vi "nanomachining test temperature.vi"() -> ()   [LabVIEW 2017]
uses:
  <vilib>/DAQmx/write.llb/DAQmx Write (Digital Bool 1Line 1Point).vi
  <vilib>/DAQmx/read.llb/DAQmx Read (Analog 1D DBL NChan 1Samp).vi
  <vilib>/DAQmx/create/channels.llb/DAQmx Create Channel (AI-Voltage-Basic).vi
  <vilib>/DAQmx/create/channels.llb/DAQmx Create Channel (DO-Digital Output).vi
  <vilib>/DAQmx/miscellaneous.llb/DAQmx Fill In Error Info.vi
  <vilib>/DAQmx/create/channels.llb/DAQmx Create Channel (AO-Voltage-Basic).vi
  <vilib>/Utility/file.llb/Write Delimited Spreadsheet (DBL).vi
  <vilib>/imath/engines/lvmath2/RunTimeEngine/Managers/WorkSpace/UID Generator.vi
  <vilib>/imath/engines/lvmath2/RunTimeEngine/RunTimeType/NIMS_RunTimeType_From StrictType (excl LVString).vi
  <instcachedir>/0/NIMS_RunTimeType_From StrictType (excl LVString)_1019F277F0A747EDBCA0F6C52CA54500.lvgen/NIMS_RunTimeType_From StrictType (excl LVString)_1019F277F0A747EDBCA0F6C52CA54500_000.vi
  <vilib>/imath/engines/lvmath2/RunTimeEngine/LocalVariableDefStatement/MC_LocalVariableDefStatement_Display.vi
  <vilib>/imath/engines/lvmath2/RunTimeEngine/Managers/SymbolTable/Clear UID.vi
  <vilib>/imath/engines/lvmath2/RunTimeEngine/NodeEndStatement/NIMS_NodeEndStatement_Output.vi
  <instcachedir>/0/NIMS_NodeEndStatement_Output_53EC0D466D134D7ABD903AC30B43404B.lvgen/NIMS_NodeEndStatement_Output_53EC0D466D134D7ABD903AC30B43404B_009.vi
  <vilib>/imath/engines/lvmath2/RunTimeEngine/ErrorHandling/NIMS_Finalize Error.vi
  <vilib>/imath/engines/lvmath2/RunTimeEngine/Managers/SymbolTable/NIMS_WorkSpace.lvlib
panel:
  in  "Stop Temperature Acquisition":bool
  in  "Pre exposure park time (msec)":u32=5000
  out "Y Park":dbl[](array[numeric])
  out "X Park":dbl[](array[numeric])
  out "Iterations areas 3":i32[](array[numeric])
  in  "Y Park (V)":dbl=10.0
  in  "X Park (V)":dbl=10.0
  in  "End exposure park time (msec)":u32=10000
  in  "Feature source file location":path
  in  "Scan Subvi-Back and Forth ?":bool
  in  "Start wait (msec)":u32=5000
  out "thermocouples (C)":dbl[](array[numeric])
  in  "Start test?":bool
  in  "Temperature control":bool
  in  "Test type":T1(tab)
  in  "Time for each line":dbl[](array[numeric])=[0.01, 0.0316, 0.1, 0.316, 1.0, 3.16, 10.0, 31.62, 100.0]
  in  "Iterations":u32=1
  in  "Line boundaries":dbl[](array[numeric])=[10.0, -10.0]
  in  "Lines position":dbl[](array[numeric])=[9.0, 8.0, 7.0, 6.0, 4.0, 1.5, -1.5, -5.0, -9.0]
  in  "Dwell time multiplication factor":dbl=1.0
  in  "Orientation":enum16{"Horizontal", "Vertical"}(ring)
  out "Lines done?":bool
  out "Iterations Lines":i32[](array[numeric])
  out "Exposure time":dbl[](array[numeric])
  out "Exposure time plus dwell time":dbl[](array[numeric])
  out "Lines done? 2":bool
  in  "Iterations 3":u32=1
  out "Exposure time 2":dbl[](array[numeric])
  out "Iterations Lines 2":i32[](array[numeric])
  out "Exposure time plus dwell time 2":dbl[](array[numeric])
  in  "Orientation 2":enum16{"Horizontal", "Vertical"}(ring)=enum."Vertical"
  in  "Dwell multiplication factor":dbl=1.0
  out "Time (sec)":dbl[](array[numeric])
  out "X (end) (V)":dbl[](array[numeric])
  out "Y (start) (V)":dbl[](array[numeric])
  out "X start (V)":dbl[](array[numeric])
  out "Y end (V)":dbl[](array[numeric])
  out "No. Pixels X":dbl[](array[numeric])
  out "No. Pixels Y":dbl[](array[numeric])
  out "Points done?":bool
  in  "Multiplicator for each instance":dbl[](array[numeric])=[0.01, 0.0316, 0.1, 0.316, 1.0, 3.16, 10.0, 31.6, 100.0]
  in  "Dwell time X factor":dbl=1.0
  in  "points X dup":dbl[](array[numeric])=[9.0, 6.0, 2.0, -3.0, -9.0, 7.5, 4.0, -0.5, -6.0]
  in  "points Y dup":dbl[](array[numeric])=[8.0, 8.0, 8.0, 8.0, 8.0, 3.0, 3.0, 3.0, 3.0]
  out "Elapsed times pointds":dbl[](array[numeric])
  out "Iterations points":i32[](array[numeric])
  out "el times 2 points":dbl[](array[numeric])
  in  "Times (s)":dbl[](array[numeric])=[0.53, 0.95, 1.69, 3.0, 5.33, 9.49, 16.87, 30.0, 53.35, 94.87, 168.7, 300.0]
  in  "Voltages y":dbl[][](array[numeric])=[[10.0, 6.0], [10.0, 6.0], [10.0, 6.0], [10.0, 6.0], [2.0, -2.0], [2.0, -2.0], [2.0, -2.0], [2.0, -2.0], [-6.0, -10.0], [-6.0, -10.0], [-6.0, -10.0], [-6.0, -10.0]]
  in  "Voltages x":dbl[][](array[numeric])=[[10.0, 7.0], [4.33, 1.33], [-1.33, -4.33], [-7.0, -10.0], [10.0, 7.0], [4.33, 1.33], [-1.33, -4.33], [-7.0, -10.0], [10.0, 7.0], [4.33, 1.33], [-1.33, -4.33], [-7.0, -10.0]]
  out "Elapsed times areas":dbl[](array[numeric])
  out "Iterations areas":i32[](array[numeric])
  out "El times areas 2":dbl[](array[numeric])
  out "Areas done?":bool
  in  "Mode":enum16{"Vertical", "Zigzag", "Horizontal"}(ring)
  in  "Freq":dbl=100000.0
  out "Elapsed Time (s)":dbl
  out "proj time":dbl
  out "Intensity Graph":dbl[][](graph)
  out "Iterations 2":i32
  in  "maxdepth":dbl=1.5
  in  "y range":dbl[](array[numeric])
  in  "x range":dbl[](array[numeric])
  in  "y pixels 2":dbl=100.0
  in  "x pixels 2":dbl=100.0
  in  "Frequency":dbl=100000.0
  out "Progress":dbl(slide) scale=0.0..1.0
  out "Dots done?":bool
  in  "Dwell time multiplicator":dbl=1.0
  out "Elapsed times points":dbl[](array[numeric])
  out "Iterations points 2":i32[](array[numeric])
  out "Loop Times points":dbl[](array[numeric])
  out "X start dots (V)":dbl[](array[numeric])
  out "Time (sec) 3":dbl[](array[numeric])
  out "Y start dots (V)":dbl[](array[numeric])
  in  "point mock frequency":dbl=10000.0 format="%#_13g"
  out "Elapsed times areas 2":dbl[](array[numeric])
  out "El times areas 3":dbl[](array[numeric])
  out "Iterations areas 2":i32[](array[numeric])
  in  "Stop Button 2":bool
  in  "Mode 2":enum16{"Vertical", "Zigzag", "Horizontal"}(ring)
  out "Line done?":bool
  in  "Dwell multiplication factor 2":dbl=0.5
  out "Time (sec) 2":dbl[](array[numeric])
  out "No. Pixels X 2":dbl[](array[numeric])
  out "No. Pixels Y 2":dbl[](array[numeric])
  out "X start (V) 2":dbl[](array[numeric])
  out "X (end) (V) 2":dbl[](array[numeric])
  out "Y (start) (V) 2":dbl[](array[numeric])
  out "Y end (V) 2":dbl[](array[numeric])
  in  "Freq 2":dbl=100000.0
  in  "Waveform Frequency":dbl=1000000.0
  in  "Area scan mode (Zigzag best)":enum16{"Vertical", "Zigzag", "Horizontal"}(ring)=enum."Zigzag"
  out "Areas done?":bool
  out "Frame Number":i32[](array[numeric])
  out "El times areas 4":dbl[](array[numeric])
  out "Elapsed times areas 3":dbl[](array[numeric])
  out "Time (s)":dbl[](array[numeric])
  in  "Dwell multiplication factor":dbl=1.0
  out "X start (V)":dbl[](array[numeric])
  out "X (end) (V)":dbl[](array[numeric])
  out "Y (start) (V)":dbl[](array[numeric])
  out "Y end (V)":dbl[](array[numeric])
  out "No. Pixels X":dbl[](array[numeric])
  out "Writing time (s)":dbl[](array[numeric])
  out "Corner dwell time (s)":dbl[](array[numeric])
  out "No. Pixels Y":dbl[](array[numeric])
  out "Autovoltage (V)":dbl
  out "thermocouples (V)":dbl[](array[numeric]) format="%0.4f"
  in  "Setpoint":dbl
  in  "Manual voltage (V)":dbl
  out "setpoint in mv":dbl
  out "I measured source":dbl format="%.2p"
  out "V source measured":dbl format="%.2p"
  out "Waveform Chart":cluster{dbl, dbl}(graph)
  in  "manual Temp. ?":bool
  in  "folder path":path
  # "automatically creates a copy on the bottom half of the screen ( negative Y)"
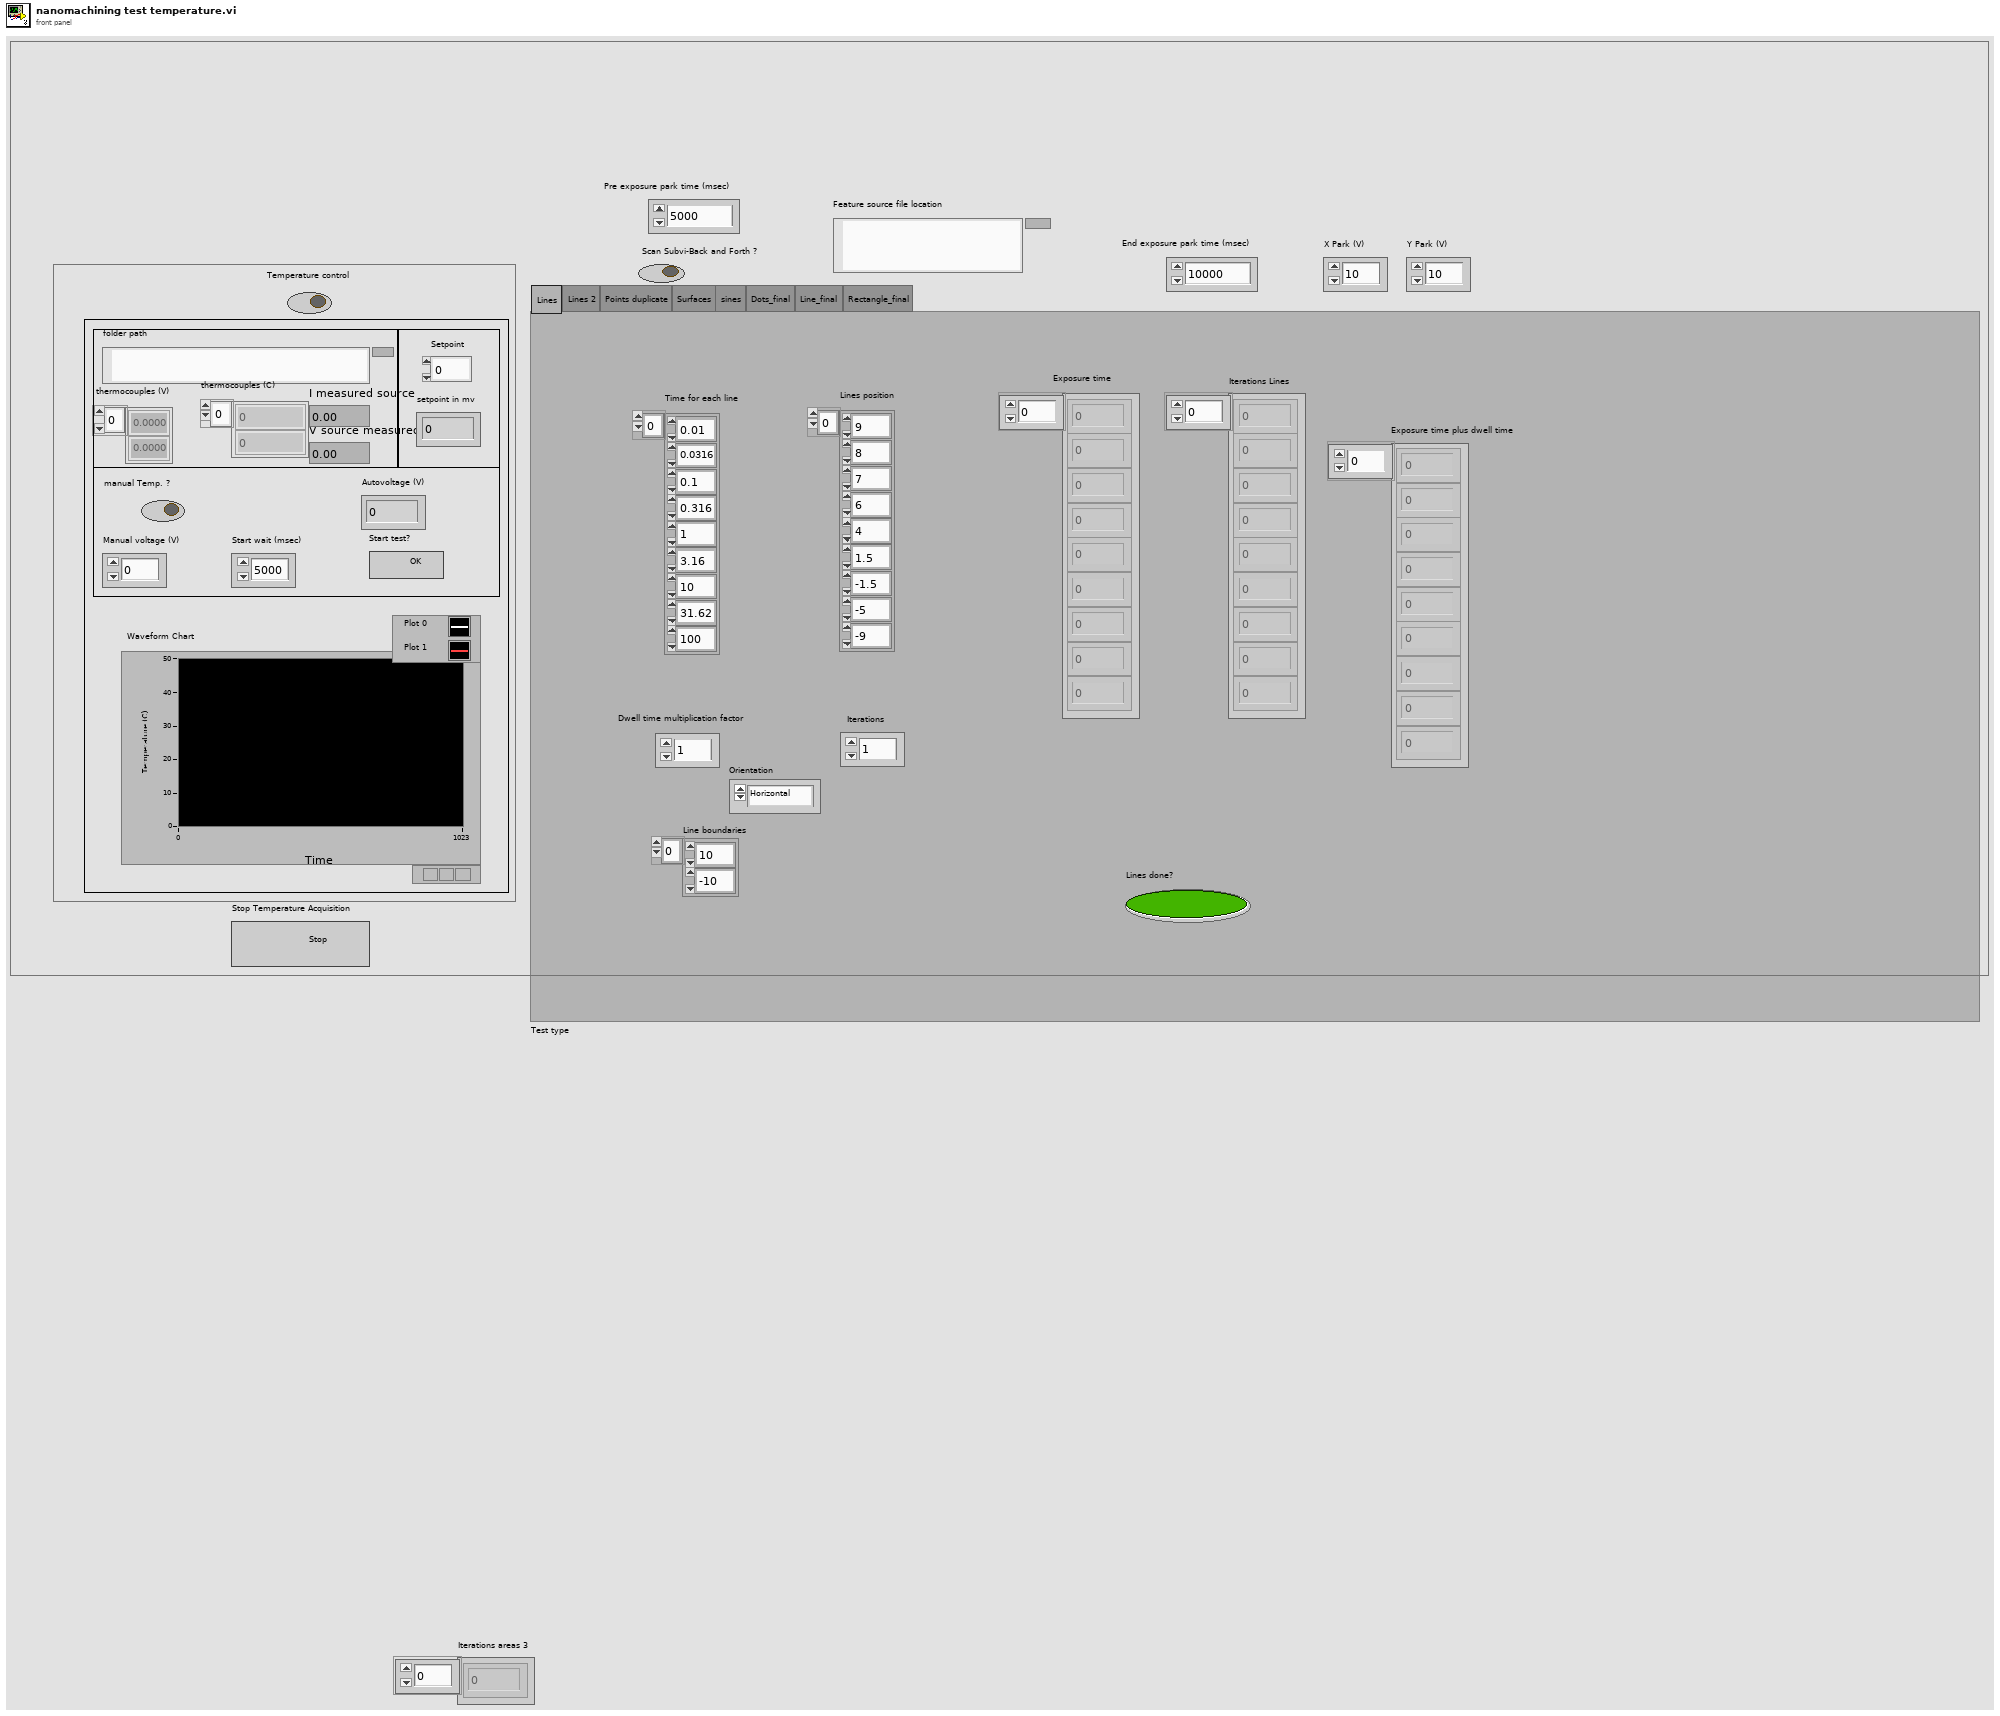
[diagram p1: front panel]
types:
  T1 = enum32{"Lines", "Lines 2", "Points duplicate", "Surfaces", "sines", "Dots_final", "Line_final", "Rectangle_final"}
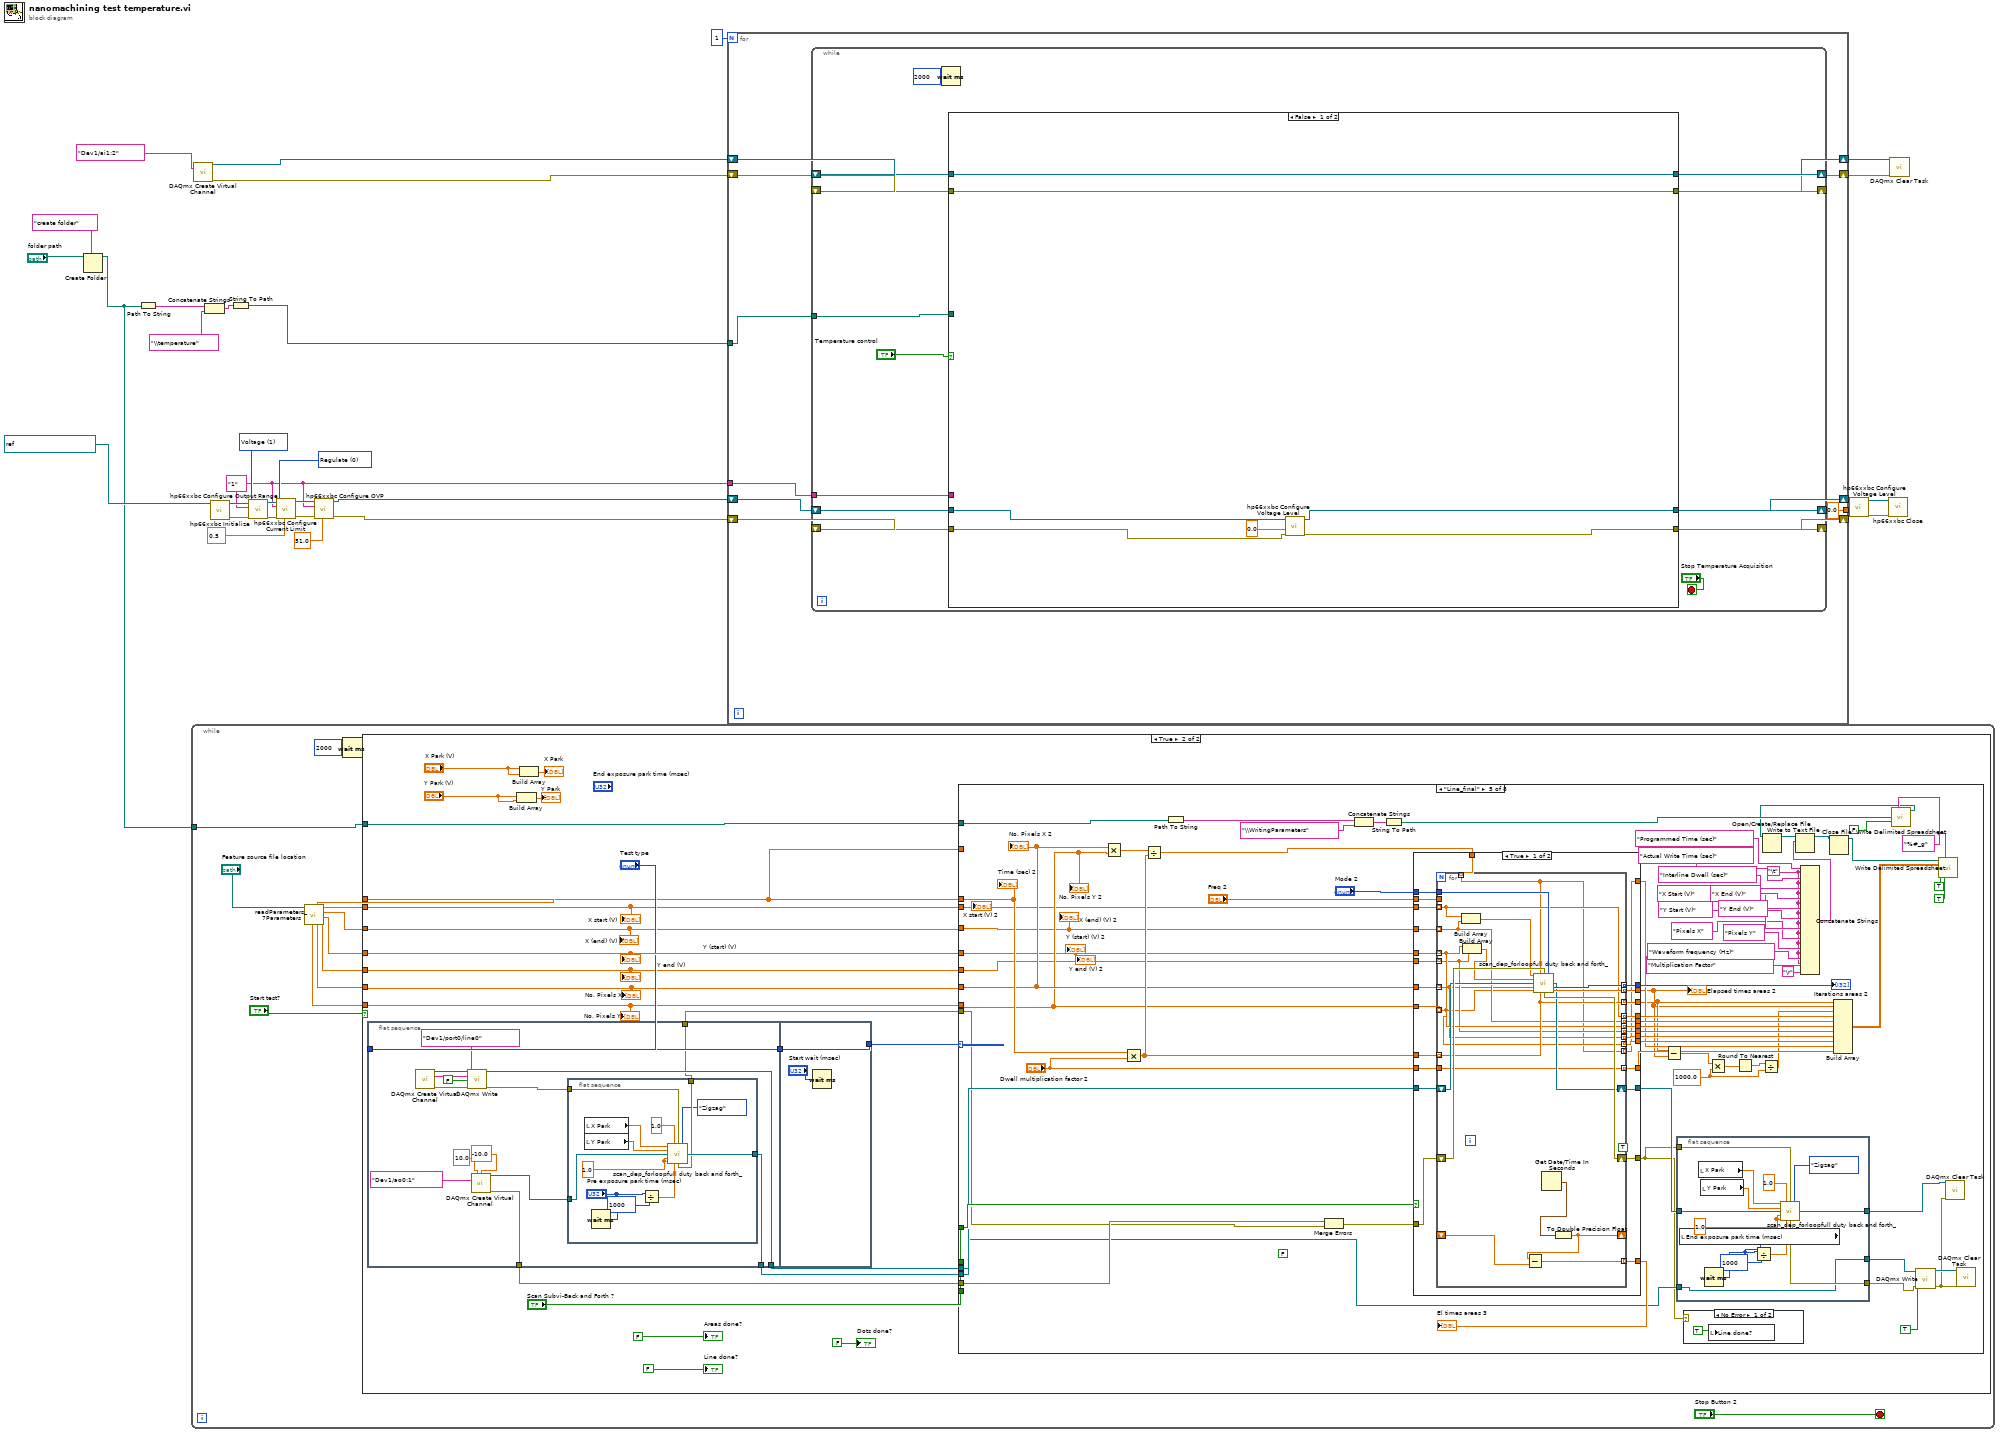
[diagram p0: block diagram]
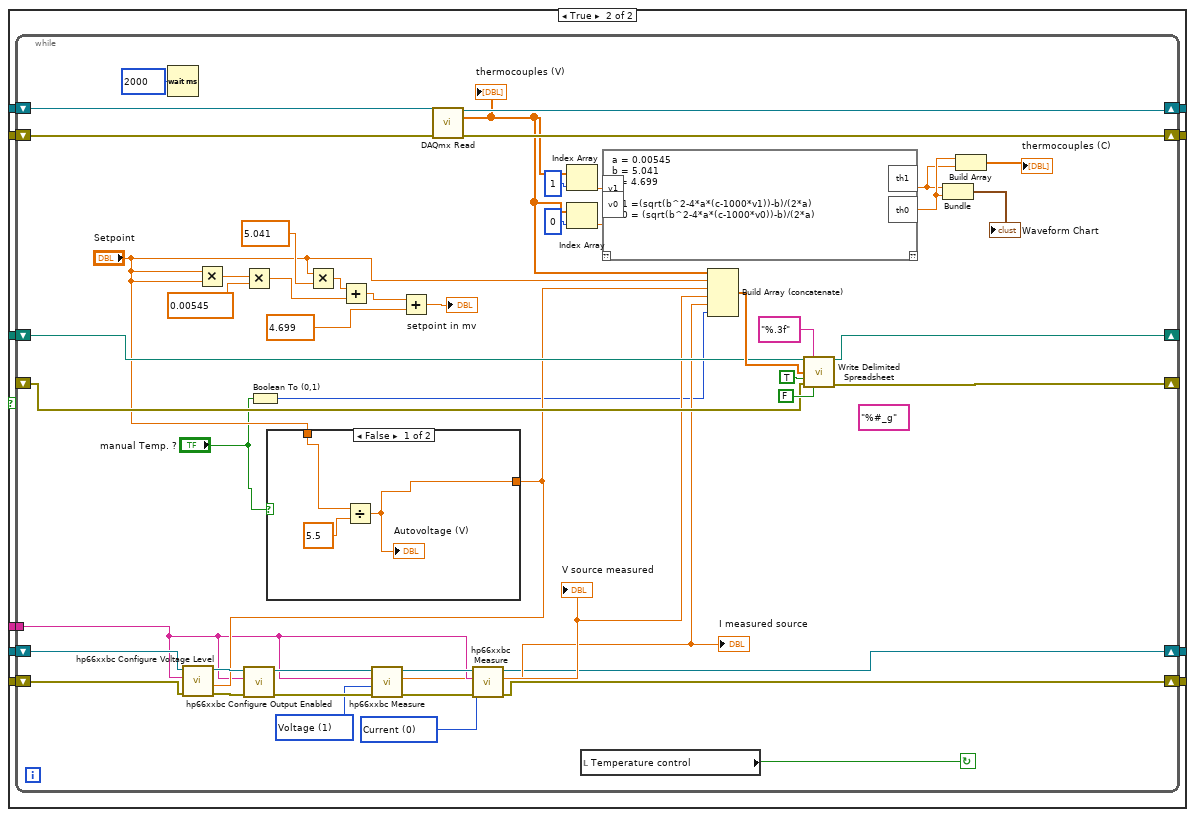
[diagram p2: hidden frame]
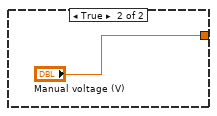
[diagram p3: hidden frame]
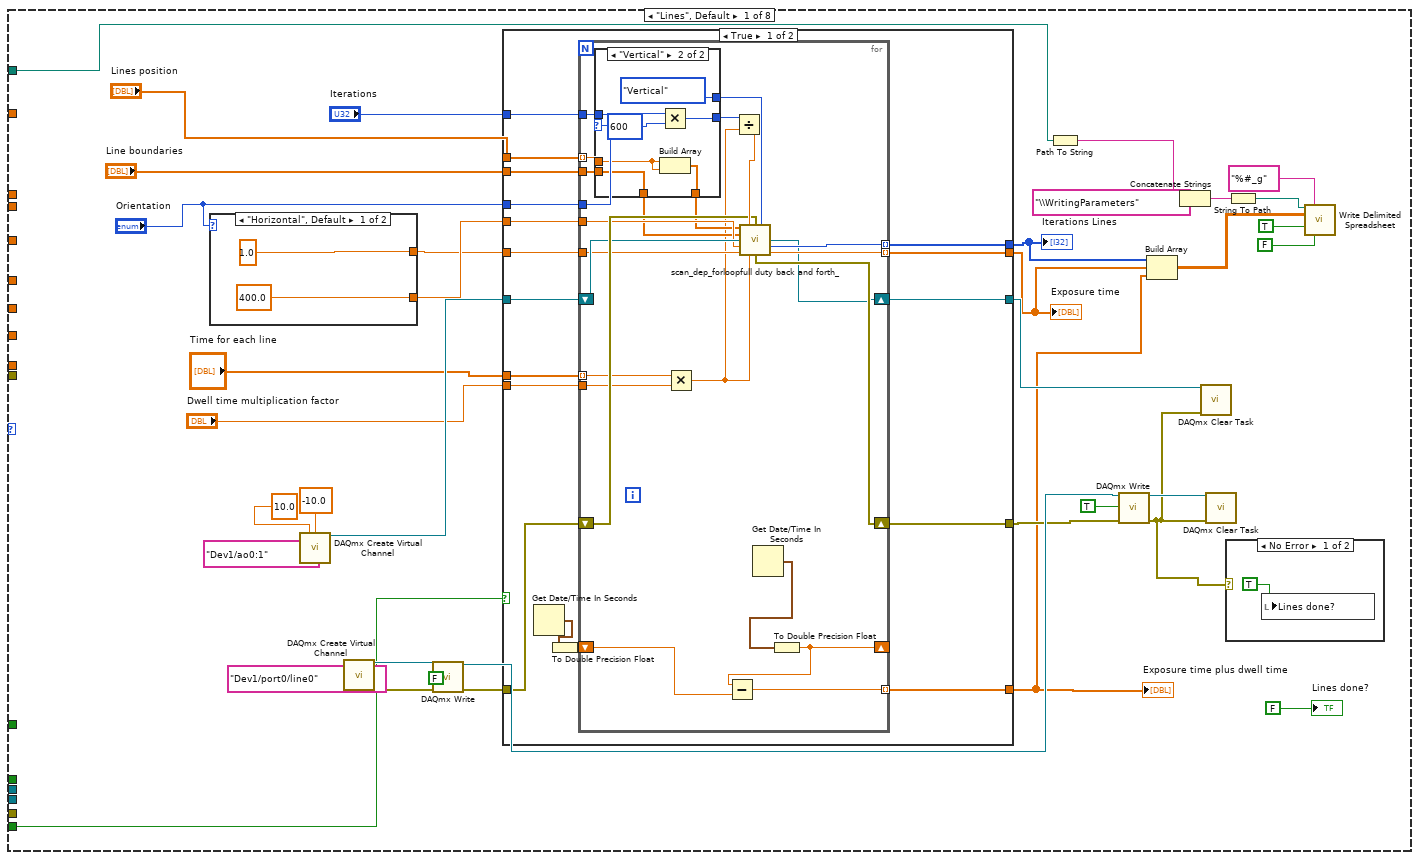
[diagram p5: hidden frame]
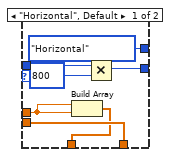
[diagram p6: hidden frame]
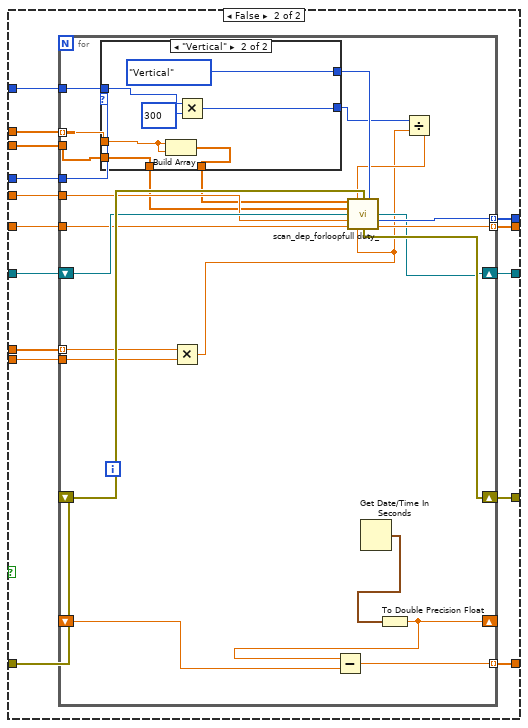
[diagram p7: hidden frame]
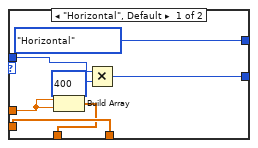
[diagram p8: hidden frame]
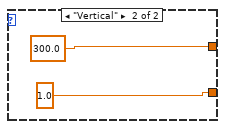
[diagram p9: hidden frame]
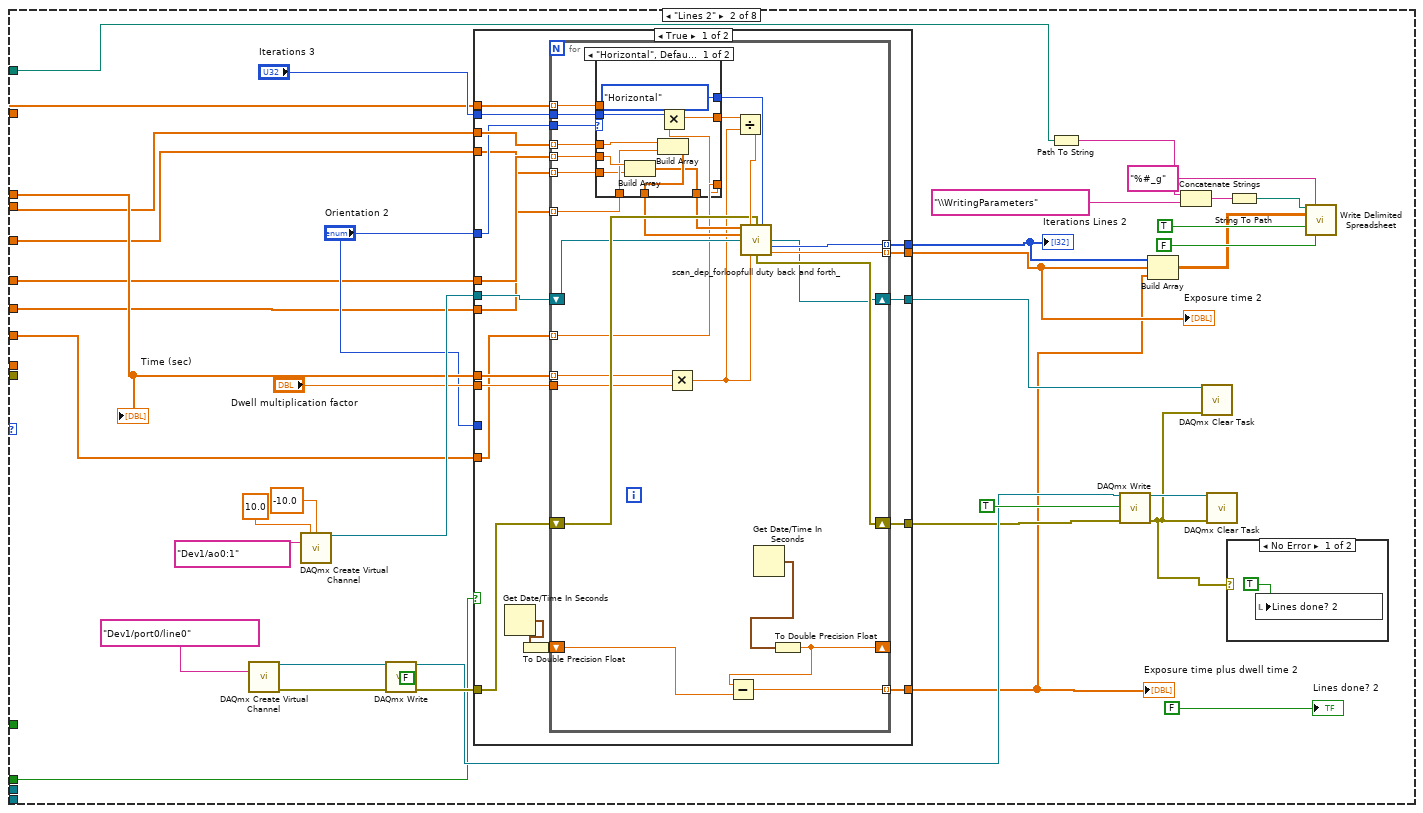
[diagram p11: hidden frame]
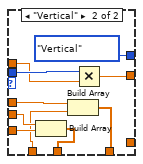
[diagram p12: hidden frame]
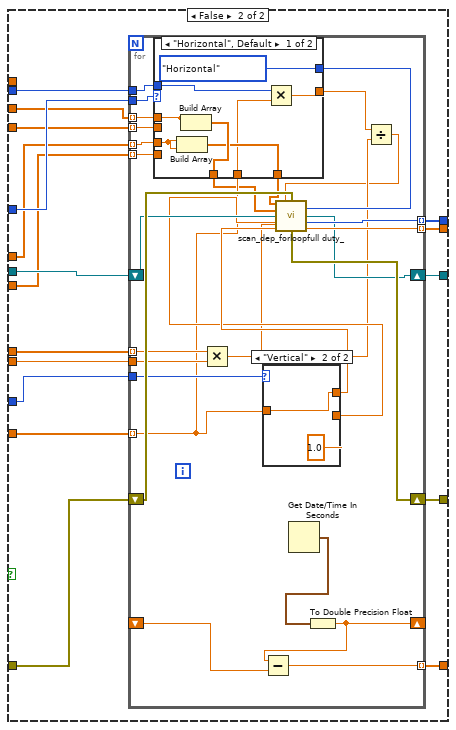
[diagram p13: hidden frame]
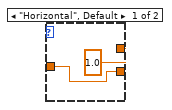
[diagram p14: hidden frame]
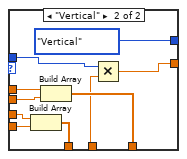
[diagram p15: hidden frame]
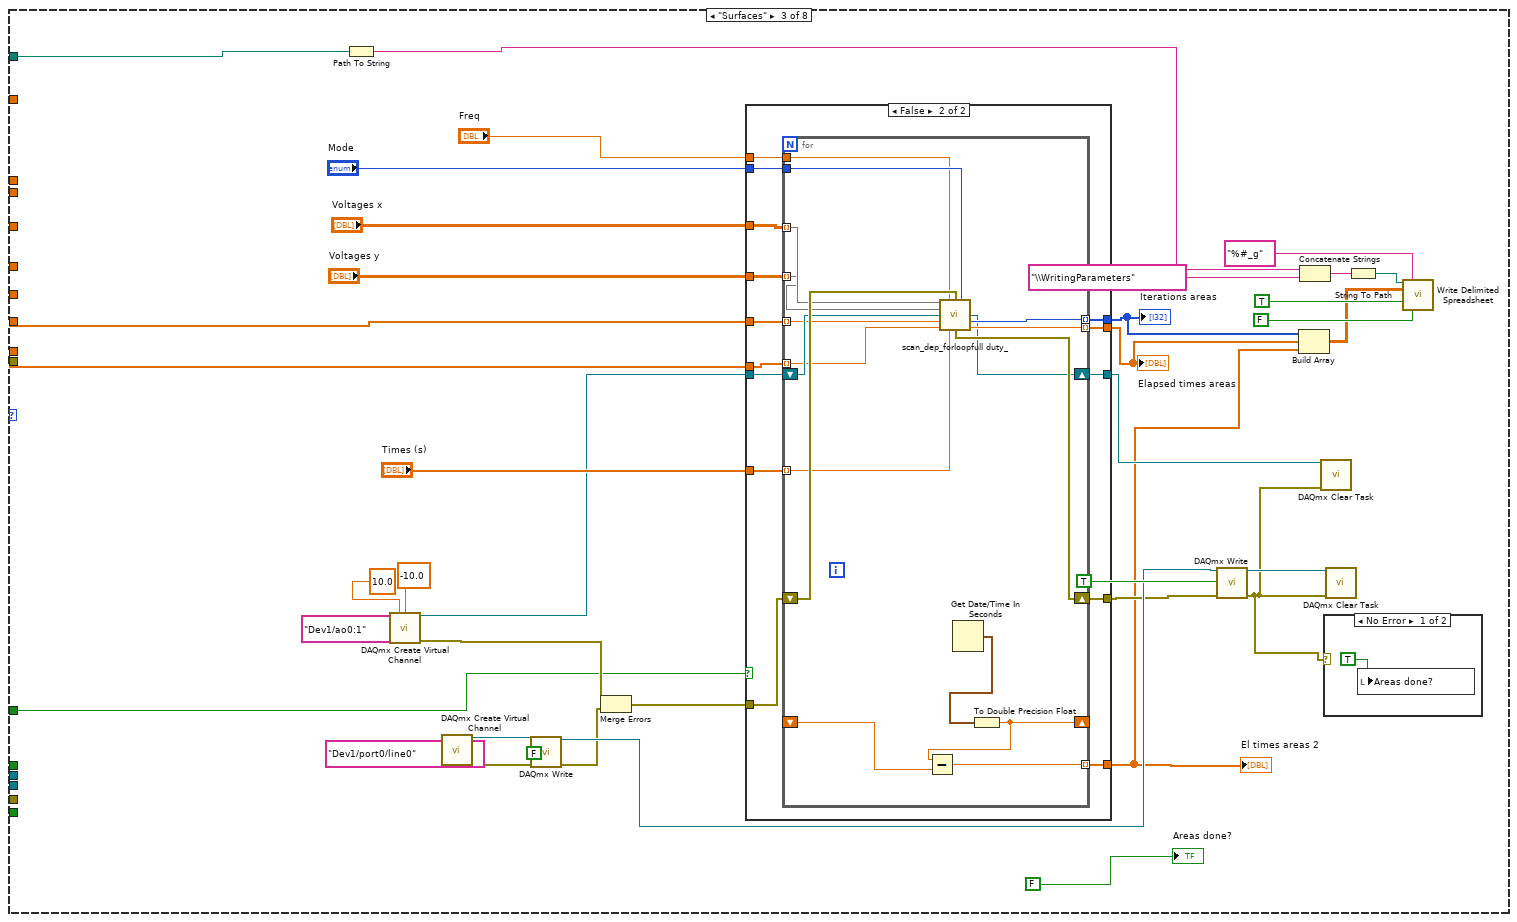
[diagram p17: hidden frame]
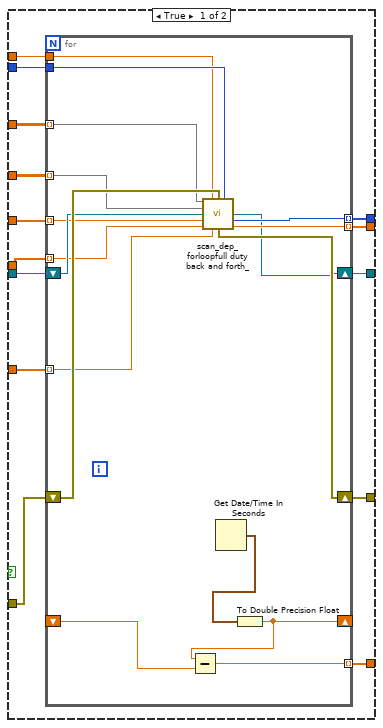
[diagram p18: hidden frame]
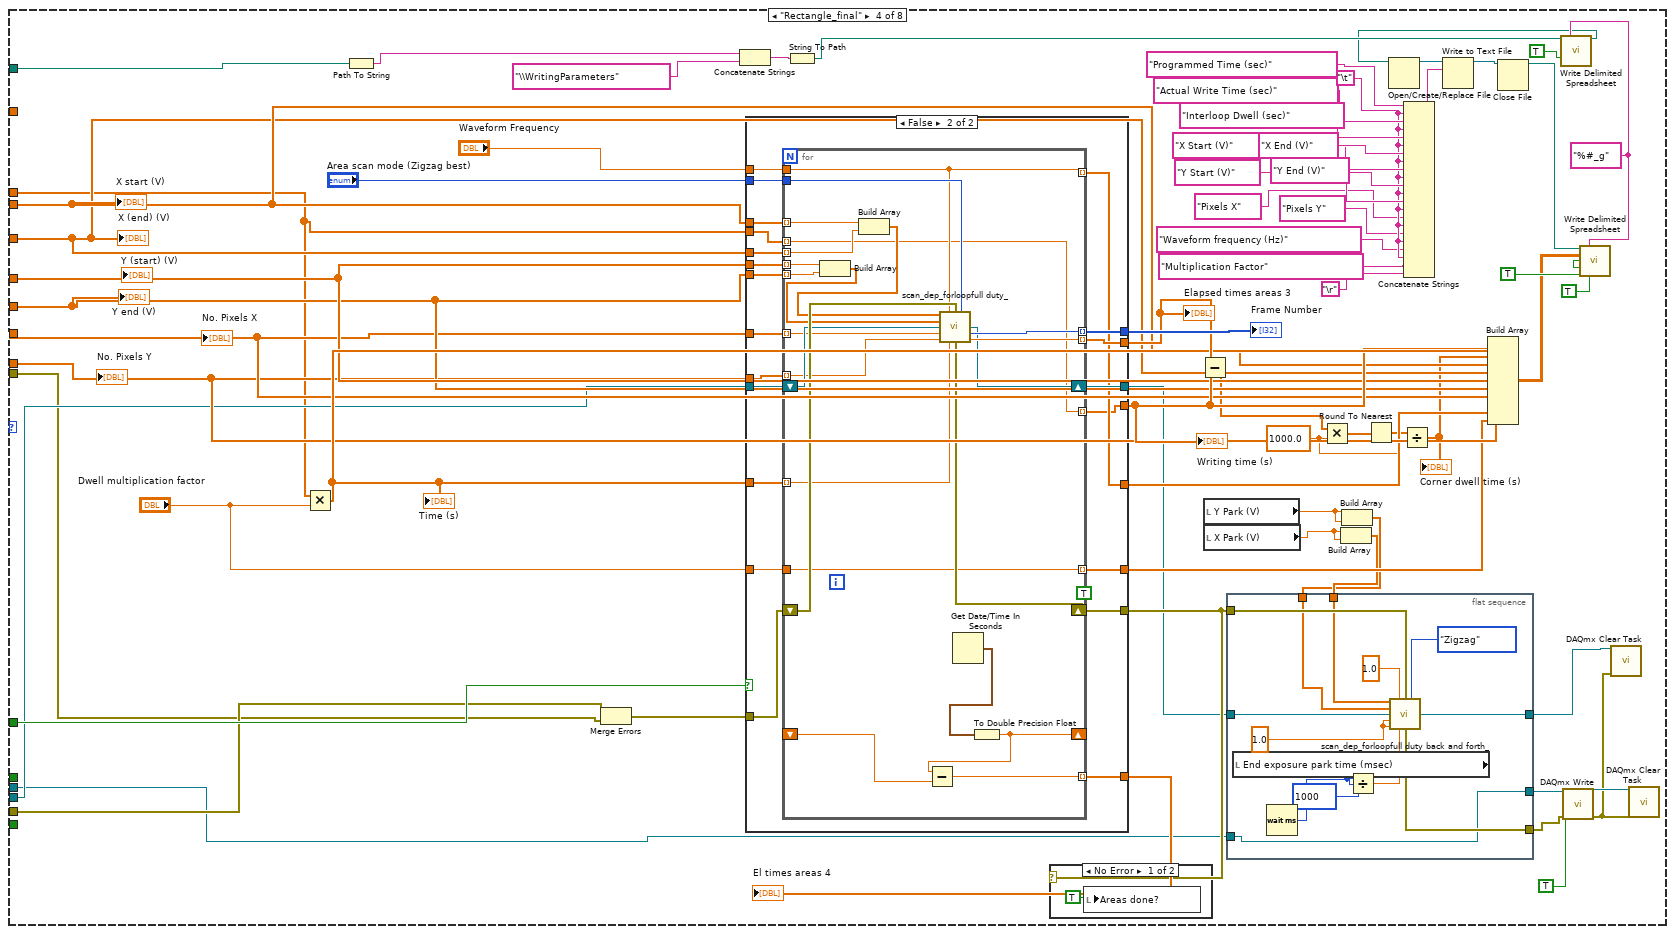
[diagram p20: hidden frame]
diagram:
  w23 = 0 items=["Regulate", "Trip"] ("behavior (0:Regulate)")
  w27 = 1 items=["Voltage"=1, "Current"=0] ("range type (1:Voltage)")
  w15 = "1" ("channel (\"\") name")
  n1 = Create Folder(prompt (Create Folder)="create folder", path (use dialog)="folder path") -> (created path=w2:path)  [unwired: 1 in, 2 out]
  n2 = Path To String(path=w2) -> (string=w9:string)
  n3 = while {
    tunnel: w2 -> [w42]
    stop <- "Stop Button 2" stop-if-true
    n4 = call "readParameters_7Parameters.vi"("file path (dialog if empty)"="Feature source file location") -> ("Y end (V)"=w37:dbl[], "Y start (V)"=w39:dbl[], "X End (V)"=w40:dbl[], "X Start (V)"=w33:dbl[], "Number Pixels X"=w36:dbl[], "Time (sec)"=w35:dbl[], "Number Pixels Y"=w34:dbl[])  [unwired: 4 in]
    n5 = Wait (ms)(milliseconds to wait=u32 2000) -> ()  [unwired: 1 out]
    n6 = case shown="True" "Start test?" {
      tunnel: w42 -> [_ w67]
      tunnel: w35 -> [_ w57]
      tunnel: w40 -> [_ w58]
      tunnel: w39 -> [_ w66]
      tunnel: w37 -> [_ w62]
      tunnel: w36 -> [_ w61]
      tunnel: w34 -> [_ w60]
      tunnel: w33 -> [_ w59]
      frame False {
      }
      frame True {
        n7 = flat-sequence {
          tunnel: "Test type" -> [w81]
          tunnel: [w81] -> w55
          tunnel: [w76] -> w54
          tunnel: [w71] -> w53
          tunnel: [w69] -> w48
          tunnel: [w68] -> w47
          tunnel: [w94] -> w64
          tunnel: w55 -> [w94]
          frame #0 {
            n8 = call-poly <vilib>:"DAQmx Create Virtual Channel.vi"("lines"=tag "Dev1/port0/line0") -> ("task out"=w79:refnum<k21>, "error out"=w80:errorcluster)  [unwired: 13 in]
            n9 = call-poly <vilib>:"DAQmx Write.vi"("task/channels in"=w79, "data"=FALSE, "error in"=w80) -> ("task out"=w76:refnum<k21>, "error out"=w72:errorcluster)  [unwired: 10 in, 1 out]
            n10 = call-poly <vilib>:"DAQmx Create Virtual Channel.vi"("maximum value"=10.0, "minimum value"=-10.0, "physical channels"=tag "Dev1/ao0:1") -> ("task out"=w70:refnum<k21>, "error out"=w68:errorcluster)  [unwired: 11 in]
            n11 = flat-sequence {
              tunnel: [w93] -> w69
              tunnel: w70 -> [w92]
              tunnel: w72 -> [w90]
              tunnel: [w89] -> w71
              frame #0 {
                w91 = 1.0 ("x pixels")
                n12 = local read "X Park"() -> (w83:dbl[])
                n13 = local read "Y Park"() -> (w82:dbl[])
                n14 = Wait (ms)(milliseconds to wait="Pre exposure park time (msec)") -> ()  [unwired: 1 out]
                n15 = Divide(x="Pre exposure park time (msec)", y=u32 1000) -> (x/y=w85:dbl)
                n16 = call "scan_dep_forloopfull duty back and forth_.vi"("x range"=w83, "Freq"=1.0, "error in"=w90, "Mode"=enum16{"Vertical", "Zigzag", "Horizontal"}."Zigzag", "y range"=w82, "task/channels in"=w92, "x pixels"=w91, "y pixels"=w91, "Time limit (s)"=w85) -> ("task out"=w93:refnum<k21>, "error IO"=w89:errorcluster)  [unwired: 2 in, 3 out]
              }
            }
          }
          frame #1 {
            n17 = Wait (ms)(milliseconds to wait="Start wait (msec)") -> ()  [unwired: 1 out]
          }
        }
        n18 = Build Array("Y Park (V)", "Y Park (V)") -> (→"Y Park":dbl[])
        n19 = Build Array("X Park (V)", "X Park (V)") -> (→"X Park":dbl[])
        n20 = case shown="\"Line_final\"" w64 {
          tunnel: w67 -> [w97 w255 w425 w575 w752 _ w886 w1001]
          tunnel: w57 -> [_ w253 _ w519 w749 _ _ w1000]
          tunnel: w59 -> [_ w252 _ w568 w743 _ _ w999]
          tunnel: w66 -> [_ w250 _ w566 w741 _ _ w998]
          tunnel: "Scan Subvi-Back and Forth ?" -> [_ w254 _ _ _ _ _ _]
          tunnel: "Scan Subvi-Back and Forth ?" -> [w96 _ _ _ _ _ _ _]
          tunnel: "Scan Subvi-Back and Forth ?" -> [_ _ w420 w573 w697 _ _ _]
          tunnel: w62 -> [_ w248 _ w565 w740 _ _ _]
          tunnel: w61 -> [_ w246 w418 w564 w747 _ _ _]
          tunnel: w60 -> [_ w247 w419 w563 w746 _ _ _]
          tunnel: w58 -> [_ w249 _ w567 w742 _ _ _]
          tunnel: w57 -> [_ _ _ _ _ _ _ _]
          tunnel: w54 -> [_ _ _ w522 w693 _ _ w955]
          tunnel: w53 -> [_ _ _ w521 w692 _ _ w954]
          tunnel: w48 -> [_ _ _ w524 w695 _ _ w953]
          tunnel: w47 -> [_ _ _ w523 w694 _ _ _]
          frame "Lines", Default {
            n21 = case shown="\"Horizontal\", Default" "Orientation" {
              tunnel: [400.0 ("y pixels") 1.0 ("x pixels")] -> w106
              tunnel: [1.0 ("x pixels") 300.0 ("y pixels")] -> w105
              frame "Horizontal", Default {
              }
              frame "Vertical" {
              }
            }
            n22 = call-poly <vilib>:"DAQmx Create Virtual Channel.vi"("maximum value"=10.0, "minimum value"=-10.0, "physical channels"=tag "Dev1/ao0:1") -> ("task out"=w125:refnum<k21>)  [unwired: 11 in, 1 out]
            n23 = call-poly <vilib>:"DAQmx Create Virtual Channel.vi"("lines"=tag "Dev1/port0/line0") -> ("task out"=w127:refnum<k21>, "error out"=w126:errorcluster)  [unwired: 13 in]
            n24 = call-poly <vilib>:"DAQmx Write.vi"("task/channels in"=w127, "data"=FALSE, "error in"=w126) -> ("task out"=w121:refnum<k21>, "error out"=w124:errorcluster)  [unwired: 10 in, 1 out]
            n25 = case shown="True" w96 {
              tunnel: w125 -> [w149 w202]
              tunnel: w124 -> [w148 w201]
              tunnel: [w147 w200] -> w120
              tunnel: [w146 w199] -> w119
              tunnel: [w145 w198] -> w112
              tunnel: [w144 w197] -> w111
              tunnel: [w143 w196] -> w110
              tunnel: w106 -> [w142 w195]
              tunnel: w105 -> [w141 w194]
              tunnel: "Time for each line" -> [w140 w193]
              tunnel: "Dwell time multiplication factor" -> [w139 w192]
              tunnel: "Line boundaries" -> [w138 w191]
              tunnel: "Lines position" -> [w137 w190]
              tunnel: "Orientation" -> [w136 w189]
              tunnel: "Iterations" -> [w135 w188]
              frame True {
                n26 = Get Date/Time In Seconds() -> (seconds since 1Jan1904=w134:timestamp)
                n27 = To Double Precision Float(number=w134) -> (double precision float=w133:dbl)
                n28 = for {
                  tunnel: [w173] -> w144 mode=indexing
                  tunnel: [w172] -> w145 mode=indexing
                  shift-right: [w170] -> w147
                  shift-left: w148 -> [w169]
                  shift-right: [w167] -> w146
                  shift-left: w149 -> [w168]
                  shift-right: [w163] -> _
                  shift-left: w133 -> [w164]
                  tunnel: [w165] -> w143 mode=indexing
                  tunnel: w142 -> [w162]
                  tunnel: w141 -> [w161]
                  tunnel: w140 -> [w160] mode=indexing
                  tunnel: w139 -> [w159]
                  tunnel: w138 -> [w158]
                  tunnel: w137 -> [w157] mode=indexing
                  tunnel: w136 -> [w156]
                  tunnel: w135 -> [w150]
                  n29 = case shown="\"Vertical\"" w156 {
                    tunnel: w158 -> [w180 w187]
                    tunnel: w157 -> [w179 w186]
                    tunnel: [w178 w187] -> w154
                    tunnel: [w180 w185] -> w155
                    tunnel: [enum16{"Vertical", "Zigzag", "Horizontal"}."Horizontal" ("Mode") enum16{"Vertical", "Zigzag", "Horizontal"}."Vertical" ("Mode")] -> w153
                    tunnel: [w175 w182] -> w152
                    tunnel: w150 -> [w174 w181]
                    frame "Horizontal", Default {
                      n30 = Build Array(w179, w179) -> (w178:dbl[])
                      n31 = Multiply(x=w174, y=u32 800) -> (x*y=w175:u32)
                    }
                    frame "Vertical" {
                      n32 = Multiply(x=w181, y=u32 600) -> (x*y=w182:u32)
                      n33 = Build Array(w186, w186) -> (w185:dbl[])
                    }
                  }
                  n34 = Multiply(x=w160, y=w159) -> (x*y=w151:dbl)
                  n35 = Divide(x=w152, y=w151) -> (x/y=w171:dbl)
                  n36 = call "scan_dep_forloopfull duty back and forth_.vi"("x range"=w155, "Freq"=w171, "error in"=w169, "Mode"=w153, "y range"=w154, "task/channels in"=w168, "x pixels"=w162, "y pixels"=w161, "Time limit (s)"=w151) -> ("task out"=w167:refnum<k21>, "Iterations"=w172:i32, "error IO"=w170:errorcluster, "Elapsed Time (s)"=w173:dbl)  [unwired: 2 in, 1 out]
                  n37 = Get Date/Time In Seconds() -> (seconds since 1Jan1904=w166:timestamp)
                  n38 = To Double Precision Float(number=w166) -> (double precision float=w163:dbl)
                  n39 = Subtract(x=w163, y=w164) -> (x-y=w165:dbl)
                }
              }
              frame False {
                n40 = for {
                  tunnel: [w226] -> w197 mode=indexing
                  tunnel: [w225] -> w198 mode=indexing
                  shift-right: [w224] -> w200
                  shift-left: w201 -> [w223]
                  shift-right: [w221] -> w199
                  shift-left: w202 -> [w222]
                  shift-right: [w217] -> _
                  shift-left: _ -> [w218]
                  tunnel: [w219] -> w196 mode=indexing
                  tunnel: w195 -> [w216]
                  tunnel: w194 -> [w215]
                  tunnel: w193 -> [w214] mode=indexing
                  tunnel: w192 -> [w213]
                  tunnel: w191 -> [w212]
                  tunnel: w190 -> [w211] mode=indexing
                  tunnel: w189 -> [w210]
                  tunnel: w188 -> [w206]
                  n41 = case shown="\"Vertical\"" w210 {
                    tunnel: w212 -> [w233 w240]
                    tunnel: w211 -> [w232 w239]
                    tunnel: [w231 w240] -> w208
                    tunnel: [w233 w238] -> w209
                    tunnel: [enum16{"Vertical", "Zigzag", "Horizontal"}."Horizontal" ("Mode") enum16{"Vertical", "Zigzag", "Horizontal"}."Vertical" ("Mode")] -> w207
                    tunnel: w206 -> [w228 w235]
                    tunnel: [w227 w234] -> w205
                    frame "Horizontal", Default {
                      n42 = Build Array(w232, w232) -> (w231:dbl[])
                      n43 = Multiply(x=w228, y=u32 400) -> (x*y=w227:u32)
                    }
                    frame "Vertical" {
                      n44 = Build Array(w239, w239) -> (w238:dbl[])
                      n45 = Multiply(x=w235, y=u32 300) -> (x*y=w234:u32)
                    }
                  }
                  n46 = Multiply(x=w214, y=w213) -> (x*y=w203:dbl)
                  n47 = Get Date/Time In Seconds() -> (seconds since 1Jan1904=w220:timestamp)
                  n48 = To Double Precision Float(number=w220) -> (double precision float=w217:dbl)
                  n49 = Subtract(x=w217, y=w218) -> (x-y=w219:dbl)
                  n50 = Divide(x=w205, y=w203) -> (x/y=w204:dbl)
                  n51 = call "scan_dep_forloopfull duty_.vi"("x range"=w209, "Freq"=w204, "error in"=w223, "Mode"=w207, "y range"=w208, "task/channels in"=w222, "x pixels"=w216, "y pixels"=w215, "Time limit (s)"=w203) -> ("task out"=w221:refnum<k21>, "Iterations"=w225:i32, "error IO"=w224:errorcluster, "Elapsed Time (s)"=w226:dbl)  [unwired: 2 in, 1 out]
                }
              }
            }
            "Exposure time" <- w111
            "Iterations Lines" <- w112
            "Exposure time plus dwell time" <- w110
            n52 = Path To String(path=w97) -> (string=w98:string)
            n53 = call-poly <vilib>:"DAQmx Write.vi"("task/channels in"=w121, "data"=TRUE, "error in"=w120) -> ("task out"=w122:refnum<k21>, "error out"=w108:errorcluster)  [unwired: 10 in, 1 out]
            n54 = Build Array(w112, w111, w110) -> (w109:dbl[][])
            n55 = Concatenate Strings(w98, "\\WritingParameters" ("string")) -> (w114:string)
            n56 = call <vilib>:"DAQmx Clear Task.vi"("task in"=w119, "error in"=w108) -> ()  [unwired: 13 in, 1 out]
            n57 = call <vilib>:"DAQmx Clear Task.vi"("task in"=w122, "error in"=w108) -> ()  [unwired: 13 in, 1 out]
            n58 = case shown="No Error" w108 {
              frame No Error {
                n59 = local write "Lines done?"(TRUE ("Points no brightness done ?")) -> ()
              }
              frame Error {
              }
            }
            n60 = String To Path(string=w114) -> (path=w113:path)
            n61 = call-poly <vilib>:"Write Delimited Spreadsheet.vi"("file path (dialog if empty)"=w113, "format (%.3f)"="%#_g", "2D data"=w109, "append to file? (new file:F)"=TRUE, "transpose? (no:F)"=FALSE) -> ()  [unwired: 9 in, 2 out]
            "Lines done?" <- FALSE ("Lines done?")
          }
          frame "Lines 2" {
            n62 = call-poly <vilib>:"DAQmx Create Virtual Channel.vi"("lines"=tag "Dev1/port0/line0") -> ("task out"=w279:refnum<k21>, "error out"=w278:errorcluster)  [unwired: 13 in]
            n63 = call-poly <vilib>:"DAQmx Create Virtual Channel.vi"("maximum value"=10.0, "minimum value"=-10.0, "physical channels"=tag "Dev1/ao0:1") -> ("task out"=w277:refnum<k21>)  [unwired: 11 in, 1 out]
            n64 = call-poly <vilib>:"DAQmx Write.vi"("task/channels in"=w279, "data"=FALSE, "error in"=w278) -> ("task out"=w273:refnum<k21>, "error out"=w276:errorcluster)  [unwired: 10 in, 1 out]
            n65 = case shown="True" w254 {
              tunnel: w277 -> [w303 w366]
              tunnel: w276 -> [w302 w365]
              tunnel: [w301 w364] -> w272
              tunnel: [w300 w363] -> w271
              tunnel: [w299 w362] -> w264
              tunnel: [w298 w361] -> w263
              tunnel: [w297 w360] -> w262
              tunnel: w253 -> [w296 w359]
              tunnel: "Dwell multiplication factor" -> [w295 w358]
              tunnel: w252 -> [w294 w352]
              tunnel: "Iterations 3" -> [w293 w357]
              tunnel: w250 -> [w290 w353]
              tunnel: "Orientation 2" -> [w289 w356]
              tunnel: "Orientation 2" -> [_ w355]
              tunnel: w246 -> [w285 w354]
              tunnel: w249 -> [w288 w351]
              tunnel: w248 -> [w287 w350]
              tunnel: w247 -> [w286 _]
              frame True {
                n66 = Get Date/Time In Seconds() -> (seconds since 1Jan1904=w292:timestamp)
                n67 = To Double Precision Float(number=w292) -> (double precision float=w291:dbl)
                n68 = for {
                  tunnel: [w329] -> w298 mode=indexing
                  tunnel: [w328] -> w299 mode=indexing
                  shift-right: [w326] -> w301
                  shift-left: w302 -> [w325]
                  shift-right: [w323] -> w300
                  shift-left: w303 -> [w324]
                  shift-right: [w319] -> _
                  shift-left: w291 -> [w320]
                  tunnel: [w321] -> w297 mode=indexing
                  tunnel: w296 -> [w318] mode=indexing
                  tunnel: w295 -> [w317]
                  tunnel: w294 -> [w316] mode=indexing
                  tunnel: w293 -> [w310]
                  tunnel: w290 -> [w309] mode=indexing
                  tunnel: w289 -> [w308]
                  tunnel: w288 -> [w307] mode=indexing
                  tunnel: w287 -> [w306] mode=indexing
                  tunnel: w286 -> [w305] mode=indexing
                  tunnel: w285 -> [w304] mode=indexing
                  n69 = case shown="\"Horizontal\", Default" w308 {
                    tunnel: w316 -> [w339 w349]
                    tunnel: [w338 w344] -> w314
                    tunnel: [w334 w348] -> w315
                    tunnel: [enum16{"Vertical", "Zigzag", "Horizontal"}."Horizontal" ("Mode") enum16{"Vertical", "Zigzag", "Horizontal"}."Vertical" ("Mode")] -> w313
                    tunnel: [w336 w346] -> w312
                    tunnel: w310 -> [w335 w345]
                    tunnel: w309 -> [w333 w343]
                    tunnel: w307 -> [w332 w340]
                    tunnel: w306 -> [w331 w342]
                    tunnel: w305 -> [_ w341]
                    tunnel: w304 -> [w330 _]
                    frame "Horizontal", Default {
                      n70 = Build Array(w333, w331) -> (w334:dbl[])
                      n71 = Build Array(w339, w332) -> (w338:dbl[])
                      n72 = Multiply(x=w335, y=w330) -> (x*y=w336:dbl)
                    }
                    frame "Vertical" {
                      n73 = Build Array(w343, w342) -> (w344:dbl[])
                      n74 = Build Array(w349, w340) -> (w348:dbl[])
                      n75 = Multiply(x=w345, y=w341) -> (x*y=w346:dbl)
                    }
                  }
                  n76 = Multiply(x=w318, y=w317) -> (x*y=w311:dbl)
                  n77 = Divide(x=w312, y=w311) -> (x/y=w327:dbl)
                  n78 = call "scan_dep_forloopfull duty back and forth_.vi"("x range"=w315, "Freq"=w327, "error in"=w325, "Mode"=w313, "y range"=w314, "task/channels in"=w324, "Time limit (s)"=w311) -> ("task out"=w323:refnum<k21>, "Iterations"=w328:i32, "error IO"=w326:errorcluster, "Elapsed Time (s)"=w329:dbl)  [unwired: 4 in, 1 out]
                  n79 = Get Date/Time In Seconds() -> (seconds since 1Jan1904=w322:timestamp)
                  n80 = To Double Precision Float(number=w322) -> (double precision float=w319:dbl)
                  n81 = Subtract(x=w319, y=w320) -> (x-y=w321:dbl)
                }
              }
              frame False {
                n82 = for {
                  tunnel: [w394] -> w361 mode=indexing
                  tunnel: [w393] -> w362 mode=indexing
                  shift-right: [w392] -> w364
                  shift-left: w365 -> [w391]
                  shift-right: [w389] -> w363
                  shift-left: w366 -> [w390]
                  shift-right: [w385] -> _
                  shift-left: _ -> [w386]
                  tunnel: [w387] -> w360 mode=indexing
                  tunnel: w359 -> [w384] mode=indexing
                  tunnel: w358 -> [w383]
                  tunnel: w352 -> [w382] mode=indexing
                  tunnel: w357 -> [w380]
                  tunnel: w355 -> [w377]
                  tunnel: w356 -> [w376]
                  tunnel: w354 -> [w375] mode=indexing
                  tunnel: w353 -> [w374] mode=indexing
                  tunnel: w351 -> [w370] mode=indexing
                  tunnel: w350 -> [w369] mode=indexing
                  n83 = case shown="\"Horizontal\", Default" w376 {
                    tunnel: w382 -> [w399 w410]
                    tunnel: [w406 w411] -> w368
                    tunnel: [w403 w416] -> w367
                    tunnel: [enum16{"Vertical", "Zigzag", "Horizontal"}."Horizontal" ("Mode") enum16{"Vertical", "Zigzag", "Horizontal"}."Vertical" ("Mode")] -> w381
                    tunnel: w380 -> [w404 w414]
                    tunnel: w374 -> [w400 w413]
                    tunnel: w375 -> [w402 w412]
                    tunnel: [w401 w409] -> w372
                    tunnel: w370 -> [_ w408]
                    tunnel: w369 -> [_ w407]
                    frame "Horizontal", Default {
                      n84 = Build Array(w400, w400) -> (w403:dbl[])
                      n85 = Build Array(w399, w399) -> (w406:dbl[])
                      n86 = Multiply(x=w404, y=w402) -> (x*y=w401:dbl)
                    }
                    frame "Vertical" {
                      n87 = Build Array(w413, w407) -> (w411:dbl[])
                      n88 = Build Array(w410, w408) -> (w416:dbl[])
                      n89 = Multiply(x=w414, y=w412) -> (x*y=w409:dbl)
                    }
                  }
                  n90 = Multiply(x=w384, y=w383) -> (x*y=w373:dbl)
                  n91 = case shown="\"Vertical\"" w377 {
                    tunnel: [w395 1.0 ("x pixels")] -> w378
                    tunnel: [1.0 ("x pixels") w397] -> w379
                    tunnel: w375 -> [w395 w397]
                    frame "Horizontal", Default {
                    }
                    frame "Vertical" {
                    }
                  }
                  n92 = Get Date/Time In Seconds() -> (seconds since 1Jan1904=w388:timestamp)
                  n93 = To Double Precision Float(number=w388) -> (double precision float=w385:dbl)
                  n94 = Subtract(x=w385, y=w386) -> (x-y=w387:dbl)
                  n95 = Divide(x=w372, y=w373) -> (x/y=w371:dbl)
                  n96 = call "scan_dep_forloopfull duty_.vi"("x range"=w367, "Freq"=w371, "error in"=w391, "Mode"=w381, "y range"=w368, "task/channels in"=w390, "x pixels"=w378, "y pixels"=w379, "Time limit (s)"=w373) -> ("task out"=w389:refnum<k21>, "Iterations"=w393:i32, "error IO"=w392:errorcluster, "Elapsed Time (s)"=w394:dbl)  [unwired: 2 in, 1 out]
                }
              }
            }
            "Exposure time 2" <- w263
            "Iterations Lines 2" <- w264
            "Exposure time plus dwell time 2" <- w262
            n97 = Path To String(path=w255) -> (string=w256:string)
            n98 = call-poly <vilib>:"DAQmx Write.vi"("task/channels in"=w273, "data"=TRUE, "error in"=w272) -> ("task out"=w274:refnum<k21>, "error out"=w260:errorcluster)  [unwired: 10 in, 1 out]
            n99 = Build Array(w264, w263, w262) -> (w261:dbl[][])
            n100 = Concatenate Strings(w256, "\\WritingParameters" ("string")) -> (w266:string)
            n101 = call <vilib>:"DAQmx Clear Task.vi"("task in"=w271, "error in"=w260) -> ()  [unwired: 13 in, 1 out]
            n102 = call <vilib>:"DAQmx Clear Task.vi"("task in"=w274, "error in"=w260) -> ()  [unwired: 13 in, 1 out]
            n103 = case shown="No Error" w260 {
              frame No Error {
                n104 = local write "Lines done? 2"(TRUE ("Points no brightness done ?")) -> ()
              }
              frame Error {
              }
            }
            n105 = String To Path(string=w266) -> (path=w265:path)
            n106 = call-poly <vilib>:"Write Delimited Spreadsheet.vi"("file path (dialog if empty)"=w265, "format (%.3f)"="%#_g", "2D data"=w261, "append to file? (new file:F)"=TRUE, "transpose? (no:F)"=FALSE) -> ()  [unwired: 9 in, 2 out]
            "Lines done? 2" <- FALSE ("Lines done?")
            "Time (sec)" <- w253
          }
          frame "Surfaces" {
            n107 = Path To String(path=w425) -> (string=w440:string)
            n108 = call-poly <vilib>:"DAQmx Create Virtual Channel.vi"("maximum value"=10.0, "minimum value"=-10.0, "physical channels"=tag "Dev1/ao0:1") -> ("task out"=w421:refnum<k21>, "error out"=w422:errorcluster)  [unwired: 11 in]
            n109 = call-poly <vilib>:"DAQmx Create Virtual Channel.vi"("lines"=tag "Dev1/port0/line0") -> ("task out"=w450:refnum<k21>, "error out"=w449:errorcluster)  [unwired: 13 in]
            n110 = call-poly <vilib>:"DAQmx Write.vi"("task/channels in"=w450, "data"=FALSE, "error in"=w449) -> ("task out"=w446:refnum<k21>, "error out"=w424:errorcluster)  [unwired: 10 in, 1 out]
            n111 = Merge Errors(w422, w424) -> (w423:errorcluster)
            n112 = case shown="False" w420 {
              tunnel: w421 -> [w469 w500]
              tunnel: [w468 w499] -> w445
              tunnel: [w467 w498] -> w444
              tunnel: [w466 w497] -> w436
              tunnel: [w465 w496] -> w435
              tunnel: [w464 w495] -> w434
              tunnel: "Times (s)" -> [w463 w494]
              tunnel: "Voltages x" -> [w462 w493]
              tunnel: "Voltages y" -> [w461 w492]
              tunnel: w419 -> [w460 w490]
              tunnel: w418 -> [w459 w491]
              tunnel: "Mode" -> [w458 w489]
              tunnel: "Freq" -> [w457 w488]
              tunnel: w423 -> [w456 w487]
              frame True {
                n113 = for {
                  tunnel: [w486] -> w465 mode=indexing
                  tunnel: [w485] -> w466 mode=indexing
                  shift-right: [w484] -> w468
                  shift-left: w456 -> [w483]
                  shift-right: [w481] -> w467
                  shift-left: w469 -> [w482]
                  shift-right: [w477] -> _
                  shift-left: _ -> [w478]
                  tunnel: [w479] -> w464 mode=indexing
                  tunnel: w463 -> [w476] mode=indexing
                  tunnel: w462 -> [w475] mode=indexing
                  tunnel: w461 -> [w474] mode=indexing
                  tunnel: w460 -> [w473] mode=indexing
                  tunnel: w459 -> [w472] mode=indexing
                  tunnel: w458 -> [w471]
                  tunnel: w457 -> [w470]
                  n114 = call "scan_dep_forloopfull duty back and forth_.vi"("x range"=w475, "Freq"=w470, "error in"=w483, "Mode"=w471, "y range"=w474, "task/channels in"=w482, "x pixels"=w472, "y pixels"=w473, "Time limit (s)"=w476) -> ("task out"=w481:refnum<k21>, "Iterations"=w485:i32, "error IO"=w484:errorcluster, "Elapsed Time (s)"=w486:dbl)  [unwired: 2 in, 1 out]
                  n115 = Get Date/Time In Seconds() -> (seconds since 1Jan1904=w480:timestamp)
                  n116 = To Double Precision Float(number=w480) -> (double precision float=w477:dbl)
                  n117 = Subtract(x=w477, y=w478) -> (x-y=w479:dbl)
                }
              }
              frame False {
                n118 = for {
                  tunnel: [w517] -> w496 mode=indexing
                  tunnel: [w516] -> w497 mode=indexing
                  shift-right: [w515] -> w499
                  shift-left: w487 -> [w514]
                  shift-right: [w508] -> _
                  shift-left: _ -> [w509]
                  tunnel: [w510] -> w495 mode=indexing
                  tunnel: w494 -> [w507] mode=indexing
                  tunnel: w493 -> [w506] mode=indexing
                  tunnel: w492 -> [w505] mode=indexing
                  tunnel: w491 -> [w504] mode=indexing
                  tunnel: w490 -> [w503] mode=indexing
                  tunnel: w489 -> [w502]
                  tunnel: w488 -> [w501]
                  shift-right: [w512] -> w498
                  shift-left: w500 -> [w513]
                  n119 = call "scan_dep_forloopfull duty_.vi"("x range"=w506, "Freq"=w501, "error in"=w514, "Mode"=w502, "y range"=w505, "task/channels in"=w513, "x pixels"=w504, "y pixels"=w503, "Time limit (s)"=w507) -> ("task out"=w512:refnum<k21>, "Iterations"=w516:i32, "error IO"=w515:errorcluster, "Elapsed Time (s)"=w517:dbl)  [unwired: 2 in, 1 out]
                  n120 = Get Date/Time In Seconds() -> (seconds since 1Jan1904=w511:timestamp)
                  n121 = To Double Precision Float(number=w511) -> (double precision float=w508:dbl)
                  n122 = Subtract(x=w508, y=w509) -> (x-y=w510:dbl)
                }
              }
            }
            "Elapsed times areas" <- w435
            "Iterations areas" <- w436
            "El times areas 2" <- w434
            n123 = call-poly <vilib>:"DAQmx Write.vi"("task/channels in"=w446, "data"=TRUE, "error in"=w445) -> ("task out"=w447:refnum<k21>, "error out"=w432:errorcluster)  [unwired: 10 in, 1 out]
            n124 = Build Array(w436, w435, w434) -> (w433:dbl[][])
            n125 = Concatenate Strings(w440, "\\WritingParameters" ("string")) -> (w438:string)
            n126 = call <vilib>:"DAQmx Clear Task.vi"("task in"=w444, "error in"=w432) -> ()  [unwired: 13 in, 1 out]
            n127 = case shown="No Error" w432 {
              frame No Error {
                n128 = local write "Areas done?"(TRUE ("Points no brightness done ?")) -> ()
              }
              frame Error {
              }
            }
            n129 = call <vilib>:"DAQmx Clear Task.vi"("task in"=w447, "error in"=w432) -> ()  [unwired: 13 in, 1 out]
            n130 = String To Path(string=w438) -> (path=w437:path)
            n131 = call-poly <vilib>:"Write Delimited Spreadsheet.vi"("file path (dialog if empty)"=w437, "format (%.3f)"="%#_g", "2D data"=w433, "append to file? (new file:F)"=TRUE, "transpose? (no:F)"=FALSE) -> ()  [unwired: 9 in, 2 out]
            "Areas done?" <- FALSE ("Lines done?")
          }
          frame "Rectangle_final" {
            w537 = "\t"
            w557 = 1000.0 ("y")
            w548 = "%#_g" ("format (%.3f)")
            (unwired) TRUE ("data")
            n132 = Multiply(x=w519, y="Dwell multiplication factor") -> (x*y=w570:dbl[])
            "Time (s)" <- w570
            n133 = Path To String(path=w575) -> (string=w583:string)
            n134 = Merge Errors(w523, w521) -> (w574:errorcluster)
            n135 = Concatenate Strings(w583, "\\WritingParameters" ("File Name: Saved Writing Parameter")) -> (w581:string)
            n136 = case shown="False" w573 {
              tunnel: w524 -> [w620 w664]
              tunnel: [w619 w663] -> w527
              tunnel: [w618 w662] -> w525
              tunnel: [w617 w661] -> w580
              tunnel: [w616 w660] -> w571
              tunnel: [w615 w659] -> w572
              tunnel: w570 -> [w614 w658]
              tunnel: w563 -> [w613 w656]
              tunnel: w564 -> [w612 w657]
              tunnel: "Area scan mode (Zigzag best)" -> [w611 w655]
              tunnel: "Waveform Frequency" -> [w610 w654]
              tunnel: w574 -> [w609 w653]
              tunnel: w568 -> [w607 w652]
              tunnel: w567 -> [w608 w651]
              tunnel: w566 -> [w606 w650]
              tunnel: w565 -> [w605 w649]
              tunnel: [w604 w645] -> w569
              tunnel: "Dwell multiplication factor" -> [w603 w647]
              tunnel: [w602 w646] -> w561
              tunnel: [w601 w648] -> w560
              tunnel: w519 -> [w600 w644]
              frame True {
                n137 = for {
                  tunnel: [w621] -> w616 mode=indexing
                  tunnel: [w643] -> w617 mode=indexing
                  shift-right: [w642] -> w619
                  shift-left: w609 -> [w641]
                  shift-right: [w639] -> w618
                  shift-left: w620 -> [w640]
                  shift-right: [w635] -> _
                  shift-left: _ -> [w636]
                  tunnel: [w637] -> w615 mode=indexing
                  tunnel: w614 -> [w634] mode=indexing
                  tunnel: w613 -> [w633] mode=indexing
                  tunnel: w612 -> [w632] mode=indexing
                  tunnel: w611 -> [w631]
                  tunnel: w610 -> [w623]
                  tunnel: w608 -> [w628] mode=indexing
                  tunnel: w607 -> [w627] mode=indexing
                  tunnel: w606 -> [w626] mode=indexing
                  tunnel: w605 -> [w625] mode=indexing
                  tunnel: [w622] -> w604 mode=indexing
                  tunnel: w603 -> [w624]
                  tunnel: [w624] -> w602 mode=indexing
                  tunnel: [w623] -> w601 mode=indexing
                  tunnel: w600 -> [w621] mode=indexing
                  n138 = Build Array(w626, w625) -> (w629:dbl[])
                  n139 = Build Array(w627, w628) -> (w630:dbl[])
                  n140 = call "scan_dep_forloopfull duty back and forth_.vi"("x range"=w630, "Freq"=w623, "error in"=w641, "Mode"=w631, "y range"=w629, "task/channels in"=w640, "x pixels"=w632, "y pixels"=w633, "Time limit (s)"=w634) -> ("task out"=w639:refnum<k21>, "Iterations"=w643:i32, "error IO"=w642:errorcluster, "Elapsed Time (s)"=w622:dbl)  [unwired: 2 in, 1 out]
                  n141 = Get Date/Time In Seconds() -> (seconds since 1Jan1904=w638:timestamp)
                  n142 = To Double Precision Float(number=w638) -> (double precision float=w635:dbl)
                  n143 = Subtract(x=w635, y=w636) -> (x-y=w637:dbl)
                }
              }
              frame False {
                n144 = for {
                  tunnel: [w687] -> w660 mode=indexing
                  tunnel: [w686] -> w661 mode=indexing
                  shift-right: [w685] -> w663
                  shift-left: w653 -> [w684]
                  shift-right: [w678] -> _
                  shift-left: _ -> [w679]
                  tunnel: [w680] -> w659 mode=indexing
                  tunnel: w658 -> [w677] mode=indexing
                  tunnel: w657 -> [w676] mode=indexing
                  tunnel: w656 -> [w675] mode=indexing
                  tunnel: w655 -> [w674]
                  tunnel: w654 -> [w667]
                  shift-right: [w682] -> w662
                  shift-left: w664 -> [w683]
                  tunnel: w652 -> [w673] mode=indexing
                  tunnel: w651 -> [w672] mode=indexing
                  tunnel: w650 -> [w669] mode=indexing
                  tunnel: w649 -> [w668] mode=indexing
                  tunnel: [w667] -> w648 mode=indexing
                  tunnel: w647 -> [w666]
                  tunnel: [w666] -> w646 mode=indexing
                  tunnel: [w665] -> w645 mode=indexing
                  tunnel: w644 -> [w665] mode=indexing
                  n145 = Build Array(w669, w668) -> (w670:dbl[])
                  n146 = Build Array(w673, w672) -> (w671:dbl[])
                  n147 = call "scan_dep_forloopfull duty_.vi"("x range"=w671, "Freq"=w667, "error in"=w684, "Mode"=w674, "y range"=w670, "task/channels in"=w683, "x pixels"=w676, "y pixels"=w675, "Time limit (s)"=w677) -> ("task out"=w682:refnum<k21>, "Iterations"=w686:i32, "error IO"=w685:errorcluster, "Elapsed Time (s)"=w687:dbl)  [unwired: 2 in, 1 out]
                  n148 = Get Date/Time In Seconds() -> (seconds since 1Jan1904=w681:timestamp)
                  n149 = To Double Precision Float(number=w681) -> (double precision float=w678:dbl)
                  n150 = Subtract(x=w678, y=w679) -> (x-y=w680:dbl)
                }
              }
            }
            "Elapsed times areas 3" <- w571
            "Frame Number" <- w580
            "El times areas 4" <- w572
            "Writing time (s)" <- w569
            n151 = String To Path(string=w581) -> (path=w549:path)
            n152 = case shown="No Error" w527 {
              frame No Error {
                n153 = local write "Areas done?"(TRUE ("Points no brightness done ?")) -> ()
              }
              frame Error {
              }
            }
            n154 = Subtract(x=w571, y=w569) -> (x-y=w556:dbl[])
            n155 = local read "Y Park (V)"() -> (w530:dbl)
            n156 = local read "X Park (V)"() -> (w531:dbl)
            n157 = flat-sequence {
              tunnel: [w599] -> w529
              tunnel: w527 -> [w597]
              tunnel: [w596] -> w528
              tunnel: w533 -> [w594]
              tunnel: w532 -> [w593]
              tunnel: w522 -> [w589]
              tunnel: [w589] -> w526
              tunnel: w525 -> [w588]
              frame #0 {
                w598 = 1.0 ("x pixels")
                n158 = local read "End exposure park time (msec)"() -> (w587:u32)
                n159 = Wait (ms)(milliseconds to wait=w587) -> ()  [unwired: 1 out]
                n160 = Divide(x=w587, y=u32 1000) -> (x/y=w591:dbl)
                n161 = call "scan_dep_forloopfull duty back and forth_.vi"("x range"=w594, "Freq"=1.0, "error in"=w597, "Mode"=enum16{"Vertical", "Zigzag", "Horizontal"}."Zigzag", "y range"=w593, "task/channels in"=w588, "x pixels"=w598, "y pixels"=w598, "Time limit (s)"=w591) -> ("task out"=w599:refnum<k21>, "error IO"=w596:errorcluster)  [unwired: 2 in, 3 out]
              }
            }
            n162 = Multiply(x=w556, y=w557) -> (x*y=w559:dbl[])
            n163 = Build Array(w531, w531) -> (w533:dbl[])
            n164 = Build Array(w530, w530) -> (w532:dbl[])
            n165 = Round To Nearest(number=w559) -> (nearest integer value=w558:dbl[])
            n166 = Divide(x=w558, y=w557) -> (x/y=w555:dbl[])
            "Corner dwell time (s)" <- w555
            n167 = Concatenate Strings("Programmed Time (sec)" ("string"), w537, "Actual Write Time (sec)" ("string"), w537, "Interloop Dwell (sec)" ("string"), w537, "X Start (V)" ("string"), w537, "X End (V)" ("string"), w537, "Y Start (V)" ("string"), w537, "Y End (V)" ("string"), w537, "Pixels X" ("string"), w537, "Pixels Y" ("string"), w537, "Waveform frequency (Hz)" ("string"), w537, "Multiplication Factor" ("string"), "\r") -> (w551:string)
            n168 = Build Array(w570, w569, w555, w568, w567, w566, w565, w564, w563, w560, w561) -> (w579:dbl[][])
            n169 = call-poly <vilib>:"Write Delimited Spreadsheet.vi"("file path (dialog if empty)"=w549, "format (%.3f)"=w548, "append to file? (new file:F)"=TRUE) -> ("new file path (Not A Path if cancelled)"=w547:path)  [unwired: 11 in, 1 out]
            n170 = Open/Create/Replace File(file path (use dialog)=w547) -> (refnum out=w554:refnum<file>)  [unwired: 5 in, 2 out]
            n171 = Write to Text File(file (use dialog)=w554, text=w551) -> (refnum out=w553:refnum<file>)  [unwired: 2 in, 2 out]
            n172 = Close File(refnum=w553) -> (path=w552:path)  [unwired: 1 in, 1 out]
            n173 = call-poly <vilib>:"DAQmx Write.vi"("task/channels in"=w526, "data"=TRUE, "error in"=w528) -> ("task out"=w586:refnum<k21>, "error out"=w578:errorcluster)  [unwired: 10 in, 1 out]
            n174 = call-poly <vilib>:"Write Delimited Spreadsheet.vi"("file path (dialog if empty)"=w552, "format (%.3f)"=w548, "2D data"=w579, "append to file? (new file:F)"=TRUE, "transpose? (no:F)"=TRUE) -> ()  [unwired: 9 in, 2 out]
            n175 = call <vilib>:"DAQmx Clear Task.vi"("task in"=w529, "error in"=w578) -> ()  [unwired: 13 in, 1 out]
            n176 = call <vilib>:"DAQmx Clear Task.vi"("task in"=w586, "error in"=w578) -> ()  [unwired: 13 in, 1 out]
            "X start (V)" <- w568
            "X (end) (V)" <- w567
            "Y (start) (V)" <- w566
            "Y end (V)" <- w565
            "No. Pixels X" <- w564
            "No. Pixels Y" <- w563
          }
          frame "Line_final" {
            w705 = 1000.0 ("y")
            w712 = "\t"
            w735 = "%#_g" ("format (%.3f)")
            (unwired) TRUE ("data")
            (unwired) FALSE ("data")
            n177 = Multiply(x=w747, y=w746) -> (x*y=w750:dbl[])
            n178 = Multiply(x=w749, y="Dwell multiplication factor 2") -> (x*y=w748:dbl[])
            n179 = Divide(x=w750, y=w748) -> (x/y=w745:dbl[])
            n180 = Path To String(path=w752) -> (string=w758:string)
            n181 = Merge Errors(w694, w692) -> (w751:errorcluster)
            n182 = Concatenate Strings(w758, "\\WritingParameters" ("string")) -> (w756:string)
            n183 = String To Path(string=w756) -> (path=w734:path)
            n184 = case shown="True" w697 {
              tunnel: w695 -> [w801 w849]
              tunnel: [w800 w848] -> w690
              tunnel: [w799 w847] -> w696
              tunnel: [w798 w846] -> w755
              tunnel: [w797 w845] -> w708
              tunnel: [w796 w844] -> w754
              tunnel: w746 -> [w795 w842]
              tunnel: w747 -> [w794 w843]
              tunnel: "Mode 2" -> [w793 w841]
              tunnel: w751 -> [w792 w840]
              tunnel: w748 -> [w791 w839]
              tunnel: w745 -> [w785 w834]
              tunnel: "Freq 2" -> [w790 _]
              tunnel: w743 -> [w789 w838]
              tunnel: w742 -> [w788 w837]
              tunnel: w741 -> [w787 w836]
              tunnel: w740 -> [w786 w835]
              tunnel: [w784 w833] -> w709
              tunnel: [w777 w832] -> w713
              tunnel: [w778 w831] -> w714
              tunnel: [w783 w830] -> w719
              tunnel: [w782 w829] -> w718
              tunnel: [w781 w828] -> w717
              tunnel: [w780 w827] -> w716
              tunnel: [w779 w826] -> w715
              tunnel: "Dwell multiplication factor 2" -> [w776 w825]
              tunnel: [w775 w824] -> w710
              frame True {
                n185 = for {
                  tunnel: [w823] -> w797 mode=indexing
                  tunnel: [w822] -> w798 mode=indexing
                  shift-right: [w821] -> w800
                  shift-left: w792 -> [w820]
                  shift-right: [w818] -> w799
                  shift-left: w801 -> [w819]
                  shift-right: [w814] -> _
                  shift-left: _ -> [w815]
                  tunnel: [w816] -> w796 mode=indexing
                  tunnel: w795 -> [w804] mode=indexing
                  tunnel: w794 -> [w805] mode=indexing
                  tunnel: w793 -> [w813]
                  tunnel: w791 -> [w810] mode=indexing
                  tunnel: w785 -> [w803] mode=indexing
                  tunnel: w790 -> [_]
                  tunnel: w789 -> [w809] mode=indexing
                  tunnel: w788 -> [w808] mode=indexing
                  tunnel: w787 -> [w807] mode=indexing
                  tunnel: w786 -> [w806] mode=indexing
                  tunnel: [w810] -> w784 mode=indexing
                  tunnel: [w809] -> w783 mode=indexing
                  tunnel: [w808] -> w782 mode=indexing
                  tunnel: [w807] -> w781 mode=indexing
                  tunnel: [w806] -> w780 mode=indexing
                  tunnel: [w805] -> w779 mode=indexing
                  tunnel: [w804] -> w778 mode=indexing
                  tunnel: [w803] -> w777 mode=indexing
                  tunnel: w776 -> [w802]
                  tunnel: [w802] -> w775 mode=indexing
                  n186 = Build Array(w809, w808) -> (w812:dbl[])
                  n187 = Build Array(w807, w806) -> (w811:dbl[])
                  n188 = call "scan_dep_forloopfull duty back and forth_.vi"("x range"=w812, "Freq"=w803, "error in"=w820, "Mode"=w813, "y range"=w811, "task/channels in"=w819, "x pixels"=w805, "y pixels"=w804, "Time limit (s)"=w810) -> ("task out"=w818:refnum<k21>, "Iterations"=w822:i32, "error IO"=w821:errorcluster, "Elapsed Time (s)"=w823:dbl)  [unwired: 2 in, 1 out]
                  n189 = Get Date/Time In Seconds() -> (seconds since 1Jan1904=w817:timestamp)
                  n190 = To Double Precision Float(number=w817) -> (double precision float=w814:dbl)
                  n191 = Subtract(x=w814, y=w815) -> (x-y=w816:dbl)
                }
              }
              frame False {
                n192 = for {
                  tunnel: [w871] -> w845 mode=indexing
                  tunnel: [w870] -> w846 mode=indexing
                  shift-right: [w869] -> w848
                  shift-left: w840 -> [w868]
                  shift-right: [w862] -> _
                  shift-left: _ -> [w863]
                  tunnel: [w864] -> w844 mode=indexing
                  tunnel: w839 -> [w858] mode=indexing
                  tunnel: w843 -> [w851] mode=indexing
                  tunnel: w842 -> [w856] mode=indexing
                  tunnel: w841 -> [w861]
                  shift-right: [w866] -> w847
                  shift-left: w849 -> [w867]
                  tunnel: w834 -> [w857] mode=indexing
                  tunnel: w838 -> [w855] mode=indexing
                  tunnel: w837 -> [w854] mode=indexing
                  tunnel: w836 -> [w853] mode=indexing
                  tunnel: w835 -> [w852] mode=indexing
                  tunnel: [w858] -> w833 mode=indexing
                  tunnel: [w857] -> w832 mode=indexing
                  tunnel: [w856] -> w831 mode=indexing
                  tunnel: [w855] -> w830 mode=indexing
                  tunnel: [w854] -> w829 mode=indexing
                  tunnel: [w853] -> w828 mode=indexing
                  tunnel: [w852] -> w827 mode=indexing
                  tunnel: [w851] -> w826 mode=indexing
                  tunnel: w825 -> [w850]
                  tunnel: [w850] -> w824 mode=indexing
                  n193 = Build Array(w855, w854) -> (w860:dbl[])
                  n194 = Build Array(w853, w852) -> (w859:dbl[])
                  n195 = call "scan_dep_forloopfull duty_reduceforLines.vi"("x range"=w860, "Freq"=w857, "error in"=w868, "Mode"=w861, "y range"=w859, "task/channels in"=w867, "x pixels"=w851, "y pixels"=w856, "Time limit (s)"=w858) -> ("task out"=w866:refnum<k21>, "Iterations"=w870:i32, "error IO"=w869:errorcluster, "Elapsed Time (s)"=w871:dbl)  [unwired: 2 in, 1 out]
                  n196 = Get Date/Time In Seconds() -> (seconds since 1Jan1904=w865:timestamp)
                  n197 = To Double Precision Float(number=w865) -> (double precision float=w862:dbl)
                  n198 = Subtract(x=w862, y=w863) -> (x-y=w864:dbl)
                }
              }
            }
            "Elapsed times areas 2" <- w708
            "Iterations areas 2" <- w755
            "El times areas 3" <- w754
            n199 = Subtract(x=w709, y=w708) -> (x-y=w703:dbl[])
            n200 = flat-sequence {
              tunnel: [w774] -> w700
              tunnel: w690 -> [w772]
              tunnel: [w771] -> w699
              tunnel: w693 -> [w766]
              tunnel: [w766] -> w698
              tunnel: w696 -> [w765]
              frame #0 {
                w773 = 1.0 ("x pixels")
                n201 = local read "End exposure park time (msec)"() -> (w762:u32)
                n202 = local read "X Park"() -> (w763:dbl[])
                n203 = local read "Y Park"() -> (w764:dbl[])
                n204 = Wait (ms)(milliseconds to wait=w762) -> ()  [unwired: 1 out]
                n205 = Divide(x=w762, y=u32 1000) -> (x/y=w768:dbl)
                n206 = call "scan_dep_forloopfull duty back and forth_.vi"("x range"=w763, "Freq"=1.0, "error in"=w772, "Mode"=enum16{"Vertical", "Zigzag", "Horizontal"}."Zigzag", "y range"=w764, "task/channels in"=w765, "x pixels"=w773, "y pixels"=w773, "Time limit (s)"=w768) -> ("task out"=w774:refnum<k21>, "error IO"=w771:errorcluster)  [unwired: 2 in, 3 out]
              }
            }
            n207 = case shown="No Error" w690 {
              frame No Error {
                n208 = local write "Line done?"(TRUE ("Points no brightness done ?")) -> ()
              }
              frame Error {
              }
            }
            n209 = Multiply(x=w703, y=w705) -> (x*y=w706:dbl[])
            n210 = Round To Nearest(number=w706) -> (nearest integer value=w707:dbl[])
            n211 = Divide(x=w707, y=w705) -> (x/y=w704:dbl[])
            n212 = Concatenate Strings("Programmed Time (sec)" ("string"), w712, "Actual Write Time (sec)" ("string"), w712, "Interline Dwell (sec)" ("string"), w712, "X Start (V)" ("string"), w712, "X End (V)" ("string"), w712, "Y Start (V)" ("string"), w712, "Y End (V)" ("string"), w712, "Pixels X" ("string"), w712, "Pixels Y" ("string"), w712, "Waveform frequency (Hz)" ("string"), w712, "Multiplication Factor" ("string"), "\r") -> (w722:string)
            n213 = Build Array(w709, w708, w704, w719, w718, w717, w716, w715, w714, w713, w710) -> (w689:dbl[][])
            n214 = call-poly <vilib>:"Write Delimited Spreadsheet.vi"("file path (dialog if empty)"=w734, "format (%.3f)"=w735, "append to file? (new file:F)"=FALSE) -> ("new file path (Not A Path if cancelled)"=w733:path)  [unwired: 11 in, 1 out]
            n215 = Open/Create/Replace File(file path (use dialog)=w733) -> (refnum out=w739:refnum<file>)  [unwired: 5 in, 2 out]
            n216 = Write to Text File(file (use dialog)=w739, text=w722) -> (refnum out=w738:refnum<file>)  [unwired: 2 in, 2 out]
            n217 = Close File(refnum=w738) -> (path=w736:path)  [unwired: 1 in, 1 out]
            n218 = call-poly <vilib>:"DAQmx Write.vi"("task/channels in"=w698, "data"=TRUE, "error in"=w699) -> ("task out"=w702:refnum<k21>, "error out"=w701:errorcluster)  [unwired: 10 in, 1 out]
            n219 = call-poly <vilib>:"Write Delimited Spreadsheet.vi"("file path (dialog if empty)"=w736, "format (%.3f)"=w735, "2D data"=w689, "append to file? (new file:F)"=TRUE, "transpose? (no:F)"=TRUE) -> ()  [unwired: 9 in, 2 out]
            n220 = call <vilib>:"DAQmx Clear Task.vi"("task in"=w700, "error in"=w701) -> ()  [unwired: 13 in, 1 out]
            n221 = call <vilib>:"DAQmx Clear Task.vi"("task in"=w702, "error in"=w701) -> ()  [unwired: 13 in, 1 out]
            "Time (sec) 2" <- w749
            "No. Pixels X 2" <- w747
            "No. Pixels Y 2" <- w746
            "X (end) (V) 2" <- w742
            "X start (V) 2" <- w743
            "Y (start) (V) 2" <- w741
            "Y end (V) 2" <- w740
          }
          frame "sines" {
            n222 = call "scan functions surfaces.vi"("Frequency"="Frequency", "maxdepth"="maxdepth", "y pixels"="y pixels 2", "x pixels"="x pixels 2", "y range"="y range", "x range"="x range") -> ("proj time"=→"proj time":dbl, "Progress"=→"Progress":dbl, "Elapsed Time (s)"=→"Elapsed Time (s)":dbl, "Iterations"=→"Iterations 2":i32, "Intensity Graph"=→"Intensity Graph":dbl[][])  [unwired: 1 in]
          }
          frame "Points duplicate" {
            n223 = Path To String(path=w886) -> (string=w894:string)
            n224 = Array Size(array="points Y dup") -> (size(s)=w920:i32)
            n225 = Build Array("points X dup", "points X dup") -> (w918:dbl[][])
            n226 = Build Array("Multiplicator for each instance", "Multiplicator for each instance") -> (w916:dbl[][])
            n227 = call-poly <vilib>:"DAQmx Create Virtual Channel.vi"("lines"=tag "Dev1/port0/line0") -> ("task out"=w907:refnum<k21>, "error out"=w906:errorcluster)  [unwired: 13 in]
            n228 = call-poly <vilib>:"DAQmx Create Virtual Channel.vi"("maximum value"=10.0, "minimum value"=-10.0, "physical channels"=tag "Dev1/ao0:1") -> ("task out"=w905:refnum<k21>)  [unwired: 11 in, 1 out]
            n229 = Initialize Array(10.0 ("element"), w920) -> (w926:dbl[])
            n230 = Subtract(x="points Y dup", y=w926) -> (x-y=w925:dbl[])
            n231 = Multiply(x=w920, y=u32 2) -> (x*y=w919:u32)
            n232 = Build Array("points Y dup", w925) -> (w917:dbl[][])
            n233 = call-poly <vilib>:"DAQmx Write.vi"("task/channels in"=w907, "data"=FALSE, "error in"=w906) -> ("task out"=w900:refnum<k21>, "error out"=w904:errorcluster)  [unwired: 10 in, 1 out]
            n234 = Multiply(x="Dwell time X factor", y=2) -> (x*y=w884:dbl)
            n235 = Reshape Array(w916, w919) -> (w915:dbl[])
            n236 = Reshape Array(w918, w919) -> (w913:dbl[])
            n237 = Reshape Array(w917, w919) -> (w914:dbl[])
            n238 = for {
              tunnel: w915 -> [w951] mode=indexing
              tunnel: w914 -> [w944] mode=indexing
              tunnel: w913 -> [w941] mode=indexing
              tunnel: w884 -> [w950]
              tunnel: [w947] -> w889 mode=indexing
              tunnel: [w946] -> w890 mode=indexing
              shift-right: [w938] -> w899
              shift-left: w904 -> [w937]
              shift-right: [w935] -> w898
              shift-left: w905 -> [w936]
              shift-right: [w931] -> _
              shift-left: _ -> [w932]
              tunnel: [w933] -> w888 mode=indexing
              n239 = Build Array(w944, w944) -> (w943:dbl[])
              n240 = Build Array(w941, w941) -> (w942:dbl[])
              n241 = Multiply(x=w951, y=w950) -> (x*y=w930:dbl)
              n242 = Divide(x=2.0, y=w930) -> (x/y=w940:dbl)
              n243 = call "scan_dep_forloopfull duty back and forth_.vi"("x range"=w942, "Freq"=w940, "error in"=w937, "Mode"=enum16{"Vertical", "Zigzag", "Horizontal"}."Zigzag", "y range"=w943, "task/channels in"=w936, "x pixels"=1.0, "y pixels"=1.0, "Time limit (s)"=w930) -> ("task out"=w935:refnum<k21>, "Iterations"=w946:i32, "error IO"=w938:errorcluster, "Elapsed Time (s)"=w947:dbl)  [unwired: 2 in, 1 out]
              n244 = Get Date/Time In Seconds() -> (seconds since 1Jan1904=w934:timestamp)
              n245 = To Double Precision Float(number=w934) -> (double precision float=w931:dbl)
              n246 = Subtract(x=w931, y=w932) -> (x-y=w933:dbl)
            }
            "Elapsed times pointds" <- w889
            "Iterations points" <- w890
            "el times 2 points" <- w888
            n247 = call-poly <vilib>:"DAQmx Write.vi"("task/channels in"=w900, "data"=TRUE, "error in"=w899) -> ("task out"=w902:refnum<k21>, "error out"=w901:errorcluster)  [unwired: 10 in, 1 out]
            n248 = Build Array(w890, w889, w888) -> (w887:dbl[][])
            n249 = Concatenate Strings(w894, "\\WritingParameters" ("string")) -> (w892:string)
            n250 = call <vilib>:"DAQmx Clear Task.vi"("task in"=w898, "error in"=w901) -> ()  [unwired: 13 in, 1 out]
            n251 = call <vilib>:"DAQmx Clear Task.vi"("task in"=w902, "error in"=w901) -> ()  [unwired: 13 in, 1 out]
            n252 = case shown="No Error" w901 {
              frame No Error {
                n253 = local write "Points done?"(TRUE ("Points no brightness done ?")) -> ()
              }
              frame Error {
              }
            }
            n254 = String To Path(string=w892) -> (path=w891:path)
            n255 = call-poly <vilib>:"Write Delimited Spreadsheet.vi"("file path (dialog if empty)"=w891, "format (%.3f)"="%#_g", "2D data"=w887, "append to file? (new file:F)"=TRUE, "transpose? (no:F)"=FALSE) -> ()  [unwired: 9 in, 2 out]
            "Points done?" <- FALSE ("Points no brightness done ?")
          }
          frame "Dots_final" {
            w967 = 1000.0 ("y")
            w971 = "\t"
            w952 = "%#_g" ("format (%.3f)")
            n256 = Path To String(path=w1001) -> (string=w1006:string)
            n257 = Concatenate Strings(w1006, "\\WritingParameters" ("string")) -> (w1004:string)
            n258 = String To Path(string=w1004) -> (path=w964:path)
            n259 = for {
              tunnel: w1000 -> [w1024] mode=indexing
              tunnel: w998 -> [w1028] mode=indexing
              tunnel: w999 -> [w1029] mode=indexing
              tunnel: "Dwell time multiplicator" -> [w1025]
              tunnel: [w1044] -> w956 mode=indexing
              tunnel: [w1043] -> w1003 mode=indexing
              shift-right: [w1039] -> w993
              shift-left: w954 -> [w1038]
              shift-right: [w1036] -> w996
              shift-left: w953 -> [w1037]
              shift-right: [w1032] -> _
              shift-left: _ -> [w1033]
              tunnel: [w1034] -> w1002 mode=indexing
              tunnel: ["point mock frequency"] -> w957 mode=indexing
              tunnel: [w1030] -> _
              tunnel: [w1030] -> _ mode=indexing
              tunnel: [w1029] -> w959 mode=indexing
              tunnel: [w1028] -> w958 mode=indexing
              tunnel: [w1027] -> w963 mode=indexing
              tunnel: [w1026] -> w962 mode=indexing
              tunnel: [w1025] -> w961 mode=indexing
              tunnel: [w1024] -> w960 mode=indexing
              (unwired) 1.0 ("y pixels")
              w1026 = 1.0 ("x pixels")
              n260 = Multiply(x=w1024, y="point mock frequency") -> (x*y=w1027:dbl)
              n261 = Build Array(w1028, w1028) -> (w1041:dbl[])
              n262 = Multiply(x=w1024, y=w1025) -> (x*y=w1030:dbl)
              n263 = Build Array(w1029, w1029) -> (w1040:dbl[])
              n264 = Get Date/Time In Seconds() -> (seconds since 1Jan1904=w1035:timestamp)
              n265 = call "scan_dep_forloopfull duty back and forth_reduceForPoints.vi"("x range"=w1040, "Freq"="point mock frequency", "error in"=w1038, "Mode"=enum16{"Vertical", "Zigzag", "Horizontal"}."Zigzag", "y range"=w1041, "task/channels in"=w1037, "x pixels"=w1026, "y pixels"=w1027, "Time limit (s)"=w1030) -> ("task out"=w1036:refnum<k21>, "Iterations"=w1043:i32, "error IO"=w1039:errorcluster, "Elapsed Time (s)"=w1044:dbl)  [unwired: 2 in, 1 out]
              n266 = To Double Precision Float(number=w1035) -> (double precision float=w1032:dbl)
              n267 = Subtract(x=w1032, y=w1033) -> (x-y=w1034:dbl)
            }
            "Elapsed times points" <- w956
            "Iterations points 2" <- w1003
            "Loop Times points" <- w1002
            n268 = case shown="No Error" w993 {
              frame No Error {
                n269 = local write "Dots done?"(TRUE ("Points no brightness done ?")) -> ()
              }
              frame Error {
              }
            }
            n270 = flat-sequence {
              tunnel: [w1022] -> w997
              tunnel: w996 -> [w1021]
              tunnel: [w1019] -> w995
              tunnel: w955 -> [w1019]
              tunnel: w993 -> [w1018]
              tunnel: [w1017] -> w994
              frame #0 {
                w1020 = 1.0 ("x pixels")
                n271 = local read "End exposure park time (msec)"() -> (w1010:u32)
                n272 = local read "X Park"() -> (w1012:dbl[])
                n273 = local read "Y Park"() -> (w1011:dbl[])
                n274 = Divide(x=w1010, y=u32 1000) -> (x/y=w1014:dbl)
                n275 = Wait (ms)(milliseconds to wait=w1010) -> ()  [unwired: 1 out]
                n276 = call "scan_dep_forloopfull duty back and forth_.vi"("x range"=w1012, "Freq"=1.0, "error in"=w1018, "Mode"=enum16{"Vertical", "Zigzag", "Horizontal"}."Zigzag", "y range"=w1011, "task/channels in"=w1021, "x pixels"=w1020, "y pixels"=w1020, "Time limit (s)"=w1014) -> ("task out"=w1022:refnum<k21>, "error IO"=w1017:errorcluster)  [unwired: 2 in, 3 out]
              }
            }
            n277 = Subtract(x=w960, y=w956) -> (x-y=w965:dbl[])
            n278 = Multiply(x=w965, y=w967) -> (x*y=w968:dbl[])
            n279 = Round To Nearest(number=w968) -> (nearest integer value=w969:dbl[])
            n280 = Divide(x=w969, y=w967) -> (x/y=w966:dbl[])
            n281 = Concatenate Strings("Programmed Time (sec)" ("string"), w971, "Actual Write Time (sec)" ("string"), w971, "Interpoint Dwell (sec)" ("string"), w971, "X Start (V)" ("string"), w971, "X End (V)" ("string"), w971, "Y Start (V)" ("string"), w971, "Y End (V)" ("string"), w971, "Pixels X" ("string"), w971, "Pixels Y" ("string"), w971, "Waveform frequency (Hz)" ("string"), w971, "Multiplication Factor" ("string"), "\r") -> (w974:string)
            n282 = Build Array(w960, w956, w966, w959, w959, w958, w958, w962, w963, w957, w961) -> (w970:dbl[][])
            n283 = call-poly <vilib>:"Write Delimited Spreadsheet.vi"("file path (dialog if empty)"=w964, "format (%.3f)"=w952, "append to file? (new file:F)"=TRUE) -> ("new file path (Not A Path if cancelled)"=w985:path)  [unwired: 11 in, 1 out]
            n284 = Open/Create/Replace File(file path (use dialog)=w985) -> (refnum out=w989:refnum<file>)  [unwired: 5 in, 2 out]
            n285 = Write to Text File(file (use dialog)=w989, text=w974) -> (refnum out=w988:refnum<file>)  [unwired: 2 in, 2 out]
            n286 = Close File(refnum=w988) -> (path=w986:path)  [unwired: 1 in, 1 out]
            n287 = call-poly <vilib>:"DAQmx Write.vi"("task/channels in"=w995, "data"=TRUE, "error in"=w994) -> ("task out"=w1008:refnum<k21>, "error out"=w1007:errorcluster)  [unwired: 10 in, 1 out]
            n288 = call-poly <vilib>:"Write Delimited Spreadsheet.vi"("file path (dialog if empty)"=w986, "format (%.3f)"=w952, "2D data"=w970, "append to file? (new file:F)"=TRUE, "transpose? (no:F)"=TRUE) -> ()  [unwired: 9 in, 2 out]
            n289 = call <vilib>:"DAQmx Clear Task.vi"("task in"=w997, "error in"=w1007) -> ()  [unwired: 13 in, 1 out]
            n290 = call <vilib>:"DAQmx Clear Task.vi"("task in"=w1008, "error in"=w1007) -> ()  [unwired: 13 in, 1 out]
            "Time (sec) 3" <- w1000
            "X start dots (V)" <- w999
            "Y start dots (V)" <- w998
          }
        }
        "Y end (V)" <- w62
        "No. Pixels X" <- w61
        "No. Pixels Y" <- w60
        "Y (start) (V)" <- w66
        "X (end) (V)" <- w58
        "X start (V)" <- w59
        "Areas done?" <- FALSE ("Lines done?")
        "Line done?" <- FALSE ("Lines done?")
        "Dots done?" <- FALSE ("Points no brightness done ?")
      }
    }
  }
  n291 = call-poly <vilib>:"DAQmx Create Virtual Channel.vi"("physical channels"=tag "Dev1/ai1:2") -> ("task out"=w3:refnum<k21>, "error out"=w30:errorcluster)  [unwired: 13 in]
  n292 = Concatenate Strings(w9, "\\temperature") -> (w7:string)
  n293 = call "hp66xxbc Initialize.vi"("resource name (\"GPIB::14::INSTR\")"=refnum<k15> "GPIB1::5::INSTR" ("resource name (\"GPIB::14::INSTR\")")) -> ("error out"=w22:errorcluster, "instrument handle"=w21:refnum<k15>)  [unwired: 9 in]
  n294 = String To Path(string=w7) -> (path=w6:path)
  n295 = call "hp66xxbc Configure Output Range.vi"("error in (no error)"=w22, "range type (1:Voltage)"=w27, "channel name (\"\")"=w15, "instrument handle"=w21) -> ("error out"=w26:errorcluster, "instrument handle out"=w25:refnum<k15>)  [unwired: 6 in]
  n296 = call "hp66xxbc Configure Current Limit.vi"("limit (0.00 A)"=0.5, "error in (no error)"=w26, "behavior (0:Regulate)"=w23, "channel name (\"\")"=w15, "instrument handle"=w25) -> ("error out"=w20:errorcluster, "instrument handle out"=w19:refnum<k15>)  [unwired: 5 in]
  n297 = call "hp66xxbc Configure OVP.vi"("limit (0.0 V)"=51.0, "error in (no error)"=w20, "channel name (\"\")"=w15, "instrument handle"=w19) -> ("error out"=w16:errorcluster, "instrument handle out"=w17:refnum<k15>)  [unwired: 6 in]
  n298 = for {
    N: 1 -> [_]
    tunnel: w15 -> [w1050]
    tunnel: [0.0 ("level (0.0)")] -> w14
    tunnel: w6 -> [w1046]
    shift-right: [w1053] -> w29
    shift-left: w30 -> [w1054]
    shift-right: [w1048] -> w11
    shift-left: w17 -> [w1052]
    shift-right: [w1047] -> w10
    shift-left: w16 -> [w1051]
    shift-right: [w1055] -> w31
    shift-left: w3 -> [w1045]
    n299 = while {
      tunnel: w1050 -> [w1062]
      tunnel: w1046 -> [w1059]
      shift-right: [w1067] -> w1055
      shift-left: w1045 -> [w1068]
      shift-right: [w1065] -> w1053
      shift-left: w1054 -> [w1066]
      shift-right: [w1061] -> w1048
      shift-left: w1052 -> [w1064]
      shift-right: [w1060] -> w1047
      shift-left: w1051 -> [w1063]
      stop <- "Stop Temperature Acquisition" stop-if-true
      n300 = Wait (ms)(milliseconds to wait=u32 2000) -> ()  [unwired: 1 out]
      n301 = case shown="False" "Temperature control" {
        tunnel: w1068 -> [w1075 w1085]
        tunnel: [w1075 w1084] -> w1067
        tunnel: w1066 -> [w1074 w1083]
        tunnel: [w1074 w1082] -> w1065
        tunnel: w1059 -> [_ w1081]
        tunnel: w1064 -> [w1072 w1080]
        tunnel: w1063 -> [w1069 w1079]
        tunnel: w1062 -> [_ w1078]
        tunnel: [w1071 w1077] -> w1061
        tunnel: [w1070 w1076] -> w1060
        frame False {
          n302 = call "hp66xxbc Configure Voltage Level.vi"("error in (no error)"=w1069, "level (0.0)"=0.0, "instrument handle"=w1072) -> ("error out"=w1070:errorcluster, "instrument handle out"=w1071:refnum<k15>)  [unwired: 7 in]
        }
        frame True {
          n303 = while {
            shift-right: [w1131] -> w1084
            shift-left: w1085 -> [w1134]
            shift-right: [w1132] -> w1082
            shift-left: w1083 -> [w1133]
            shift-right: [w1126] -> _
            shift-left: _ -> [w1125]
            shift-right: [w1124] -> _
            shift-left: w1081 -> [w1123]
            shift-right: [w1098] -> w1076
            shift-left: w1079 -> [w1110]
            shift-right: [w1097] -> w1077
            shift-left: w1080 -> [w1111]
            tunnel: w1078 -> [w1102]
            stop <- w1091 continue-if-true
            (unwired) "%#_g" ("format (%.3f)")
            w1103 = 0 items=["Voltage"=1, "Current"=0] ("measurement type (1:voltage)")
            w1106 = 1 items=["Voltage"=1, "Current"=0] ("measurement type (1:voltage)")
            n304 = Wait (ms)(milliseconds to wait=u32 2000) -> ()  [unwired: 1 out]
            n305 = Multiply(x="Setpoint", y="Setpoint") -> (x*y=w1122:dbl)
            n306 = Multiply(x=w1122, y=0.00545) -> (x*y=w1119:dbl)
            n307 = Boolean To (0,1)(Boolean="manual Temp. ?") -> (0, 1=w1089:i16)
            n308 = case shown="False" "manual Temp. ?" {
              tunnel: [w1262 "Manual voltage (V)"] -> w1109
              tunnel: "Setpoint" -> [w1263 _]
              frame False {
                n309 = Divide(x=w1263, y=5.5) -> (x/y=w1262:dbl)
                "Autovoltage (V)" <- w1262
              }
              frame True {
              }
            }
            n310 = call "hp66xxbc Configure Voltage Level.vi"("error in (no error)"=w1110, "level (0.0)"=w1109, "channel name (\"\")"=w1102, "instrument handle"=w1111) -> ("error out"=w1113:errorcluster, "instrument handle out"=w1112:refnum<k15>)  [unwired: 6 in]
            n311 = call "hp66xxbc Configure Output Enabled.vi"("error in (no error)"=w1113, "channel (\"\") name"=w1102, "instrument handle"=w1112) -> ("error out"=w1107:errorcluster, "instrument handle out"=w1108:refnum<k15>)  [unwired: 7 in]
            n312 = Multiply(x="Setpoint", y=5.041) -> (x*y=w1120:dbl)
            n313 = Add(x=w1120, y=w1119) -> (x+y=w1117:dbl)
            n314 = call "hp66xxbc Measure.vi"("error in (no error)"=w1107, "measurement type (1:voltage)"=w1106, "channel name (\"\")"=w1102, "instrument handle"=w1108) -> ("error out"=w1105:errorcluster, "measurement"=w1101:dbl, "instrument handle out"=w1104:refnum<k15>)  [unwired: 5 in]
            "V source measured" <- w1101
            n315 = Add(x=w1117, y=4.699) -> (x+y=→"setpoint in mv":dbl)
            n316 = call-poly <vilib>:"DAQmx Read.vi"("task/channels in"=w1134, "error in"=w1133) -> ("task out"=w1131:refnum<k21>, "data"=w1095:dbl[], "error out"=w1132:errorcluster)  [unwired: 11 in]
            "thermocouples (V)" <- w1095
            n317 = call "hp66xxbc Measure.vi"("error in (no error)"=w1105, "measurement type (1:voltage)"=w1103, "channel name (\"\")"=w1102, "instrument handle"=w1104) -> ("error out"=w1098:errorcluster, "measurement"=w1100:dbl, "instrument handle out"=w1097:refnum<k15>)  [unwired: 5 in]
            "I measured source" <- w1100
            n318 = Index Array(array=w1095, index=1) -> (element=w1093:dbl)
            n319 = Index Array(array=w1095, index=0) -> (element=w1094:dbl)
            n320 = local read "Temperature control"() -> (w1091:bool)
            n321 = mathscript code="a = 0.00545\nb = 5.041\nc = 4.699\n\nth1 =(sqrt(b^2-4*a*(c-1000*v1))-b)/(2*a)\nth0 = (sqrt(b^2-4*a*(c-1000*v0))-b)/(2*a)"("v1"=w1093, "v0"=w1094) -> ("th0"=w1088:cdb, "th1"=w1087:cdb)  [unwired: 1 in, 1 out]
            n322 = Build Array (concatenate)(w1095, "Setpoint", w1109, w1101, w1100, w1089) -> (w1127:dbl[])
            n323 = call-poly <vilib>:"Write Delimited Spreadsheet.vi"("file path (dialog if empty)"=w1123, "format (%.3f)"="%.3f", "1D data"=w1127, "append to file? (new file:F)"=TRUE, "error in (no error)"=w1125, "transpose? (no:F)"=FALSE) -> ("new file path (Not A Path if cancelled)"=w1124:path, "error out"=w1126:errorcluster)  [unwired: 8 in]
            n324 = Bundle("th1"=w1087, "th0"=w1088) -> (→"Waveform Chart":cluster{"th1":cdb, "th0":cdb})  [unwired: 1 in]
            n325 = Build Array(w1088, w1087) -> (→"thermocouples (C)":cdb[])
          }
        }
      }
    }
  }
  n326 = call "hp66xxbc Configure Voltage Level.vi"("error in (no error)"=w10, "level (0.0)"=w14, "instrument handle"=w11) -> ("error out"=w13:errorcluster, "instrument handle out"=w12:refnum<k15>)  [unwired: 7 in]
  n327 = call "hp66xxbc Close.vi"("error in (no error)"=w13, "instrument handle"=w12) -> ()  [unwired: 9 in, 1 out]
  n328 = call <vilib>:"DAQmx Clear Task.vi"("task in"=w31, "error in"=w29) -> ()  [unwired: 13 in, 1 out]
